vi "POM_PROM_host.vi"() -> ()   [LabVIEW 2013]
uses:
  <instrlib>/niDMM/nidmm.llb/niDMM Resolution in Digits.ctl
  <instrlib>/niDMM/nidmm.llb/niDMM Function.ctl
  <instrlib>/niDCPower/nidcpower.llb/niDCPower Measurement Type.ctl
  <vilib>/Analysis/baseanly.llb/Mean (DBL).vi
  <instrlib>/niDMM/nidmm.llb/niDMM Configure Measurement Digits.vi
  <vilib>/Analysis/NI_AALBase.lvlib
panel:
  in  "Без Офира":bool
  in  "Полярность":bool
  out "Optical Power":dbl(graph)
  out "Operating Current":dbl(graph)=49.97619998441659
  in  "№#":i16=2004
  out "Стабилизировано":bool=TRUE
  in  "+ V TEC для новой точки":dbl=0.11 format="%#_13g"
  in  "Вычет для \"антиразгона\"":dbl format="%#_13g"
  in  "Оставить в раб.\nрежиме":bool
  out "Boolean":bool
  in  "Num_hits_req":u64=5
  out "Num_hits":u64=6
  in  "Count_hits?":bool
  in  "tstab между точками, мс":u32=1
  in  "Предел тока PDext, мА":dbl=20.0
  in  "Dose":i32=1
  in  "Отладка(F)/\n/Рабочий(T)":bool=TRUE
  out "TEC_current, mA":dbl=91.96261106356566
  out "V2(Ild)_Log_address":refnum<file>
  out "Ipd(Ild)_External_Log_address":refnum<file>
  in  "Param_Log":path=path "D:/#rkm/Испытания/Фонон-4/ТермоЛазер/Фонон-4_ПОМ_ПрОМ/Прога/Updated/ThermoLaser/Logs/Добор дозы"
  out "Param_Log_address":refnum<file>
  out "Op(Ild)_Log_address":refnum<file>
  out "Ipd(Ild)_Monitor_Log_address":refnum<file>
  in  "trelax":u32=35000
  out "Volt_onRes":dbl=2.704172165675047
  out "NoStab":bool
  out "Operating Current, mA":dbl=49.97619998441659
  in  "Desirable Operating current, mA":dbl=50.0 format="%#_6f"
  out "Error message":string
  in  "Up_Volt_limit":dbl=5.0
  in  "Low_Volt_limit":dbl=1.0
  out "ThRes_stabil":bool=TRUE
  out "Подстроенное напряжение\nстабилизации":dbl=0.23473322916666667
  out "ThRes value":dbl=17940.031640625
  in  "Optimum ThRes":dbl=18000.0 format="%#_6f"
  in  "Предел тока LD, мА":dbl=80.0
  in  "Предел тока ТЕС, мА":dbl=300.0
  in  "Tab Control":enum32{"Page 1", "Page 2", "Page 3", "Page 4"}(tab)=enum."Page 4"
  out "RES(U_TEC) Graph":cluster{dbl[], dbl[]}(graph)={[-0.0, 0.025, 0.05, 0.07500000000000001, 0.1, 0.125, 0.15, 0.175, 0.19999999999999998, 0.22499999999999998, 0.24999999999999997, 0.27499999999999997, 0.3, 0.325, 0.35000000000000003, 0.37500000000000006, 0.4000000000000001, 0.4250000000000001, 0.4500000000000001, 0.47500000000000014, 0.5000000000000001, 0.5250000000000001, 0.5500000000000002, 0.5750000000000002, 0.6000000000000002, 0.6250000000000002, 0.6500000000000002, 0.6750000000000003, 0.7000000000000003, 0.7250000000000003, 0.7500000000000003, 0.7750000000000004], [15319.04365234375, 15328.19267578125, 15358.49169921875, 15409.562109375, 15479.3826171875, 15563.1861328125, 15668.50888671875, 15780.12734375, 15906.40224609375, 16043.244921875, 16186.97255859375, 16341.84609375, 16507.0697265625, 16676.522265625, 16856.963671875, 17044.884375, 17239.0294921875, 17436.3736328125, 17641.744140625, 17850.8728515625, 18071.7896484375, 18291.20625, 18518.965625, 18750.4271484375, 18987.4517578125, 19230.0744140625, 19480.026171875, 19731.8517578125, 19984.940234375, 20249.54140625, 20514.206640625, 20780.055078125]}
  out "RES(I_TEC) Graph":cluster{dbl[], dbl[]}(graph)={[0.03457500435386299, 4.049114950716204, 7.9212407853678135, 11.611043015146826, 15.078954849250364, 18.53827902856892, 21.88408259580828, 25.295266856430793, 28.546483256934756, 31.60504570629327, 34.77027313644012, 37.80993408960394, 40.856486299311584, 43.94949565069024, 47.03219408159836, 50.06845592920464, 52.92926046093485, 55.95350027659507, 58.865931959242474, 61.84202368829837, 64.7802788203752, 67.60156326899994, 70.44177990185035, 73.41963022613506, 76.46974363403558, 79.22741287887104, 82.2001312992484, 85.07135997639818, 88.0785044464861, 90.98931976346292, 93.95691599392462, 96.75420696595256], [15319.04365234375, 15328.19267578125, 15358.49169921875, 15409.562109375, 15479.3826171875, 15563.1861328125, 15668.50888671875, 15780.12734375, 15906.40224609375, 16043.244921875, 16186.97255859375, 16341.84609375, 16507.0697265625, 16676.522265625, 16856.963671875, 17044.884375, 17239.0294921875, 17436.3736328125, 17641.744140625, 17850.8728515625, 18071.7896484375, 18291.20625, 18518.965625, 18750.4271484375, 18987.4517578125, 19230.0744140625, 19480.026171875, 19731.8517578125, 19984.940234375, 20249.54140625, 20514.206640625, 20780.055078125]}
  out "I_PD_Ext(I_LD) Graph":cluster{dbl[], dbl[]}(graph)={[0.0, 5.125820672560687, 10.202363077068034, 15.09070291650038, 20.026524721844005, 24.848748653112324, 29.706585438813228, 34.55255888002156, 39.41379829521783, 44.31743313126964, 49.35841653002704], [0.6213749657825949, 0.6126206411732633, 0.5986137214569519, 0.5846068013204628, 0.5933611264550083, 0.5670981505590477, 0.5355825775341941, 0.586357666360488, 0.5355825775341941, 0.5478386339632713, 0.5390843079753067]}
  out "I_PD(I_LD) Graph":cluster{dbl[], dbl[]}(graph)={[0.0, 5.125820672560687, 10.202363077068034, 15.09070291650038, 20.026524721844005, 24.848748653112324, 29.706585438813228, 34.55255888002156, 39.41379829521783, 44.31743313126964, 49.35841653002704], [0.00446055423708458, 0.1890051237296575, 1.3185992656872259, 47.69851657329127, 96.3842059718445, 145.3466946259141, 195.95923949964345, 243.1108383461833, 288.08951028622687, 334.6654470078647, 377.8655605856329]}
  out "I_pd, uA":dbl
  out "IPD(ext), mA":dbl
  out "V2(I_LD) Graph":cluster{dbl[], dbl[]}(graph)={[0.0, 5.125820672560687, 10.202363077068034, 15.09070291650038, 20.026524721844005, 24.848748653112324, 29.706585438813228, 34.55255888002156, 39.41379829521783, 44.31743313126964, 49.35841653002704], [0.0006418486043783589, 1.1699665507043246, 1.452329111789965, 1.6798119558569469, 1.9201177244634586, 2.150803801269446, 2.3862573437846697, 2.612869753183121, 2.8439823589319366, 3.0683008415602466, 3.3013683877429134]}
  out "Forward Voltage, V":dbl
  out "OP(I_LD) Graph":cluster{dbl[], dbl[]}(graph)={[0.0, 5.125820672560687, 10.202363077068034, 15.09070291650038, 20.026524721844005, 24.848748653112324, 29.706585438813228, 34.55255888002156, 39.41379829521783, 44.31743313126964, 49.35841653002704], [0.0, 0.0, 0.02, 0.74, 1.5, 2.27, 3.0300000000000002, 3.8, 4.58, 5.33, 6.119999999999999]}
  out "Ophir, mW":dbl
  out "Пороговый ток":dbl
  out "Boolean 2":bool
  out "Сопротивление терморез-ра":dbl(graph)=16035.80078125
  out "thRes_adj":dbl=16035.80078125 format="%0.2f"
  in  "Source-Ohm w8":u32=1000
  in  "Coeff_High":dbl=90000.0 format="%#_13g"
  in  "Coeff_low":dbl=20000.0 format="%#_13g"
  in  "Coeff_thr":dbl=1500.0
  out "+Voltage\nrequired":dbl=0.0008410915798611111
  out "Разница ThRes":dbl=75.6982421875
  out "IPD_ext, mA":dbl(graph)=16035.80078125
  out "accommodated voltage (out)":dbl=5.970992601042338
  in  "4070_Rele_source":enum16{"S2_Ch0", "S1_Ch2"}(ring)
  in  "the upper limit for the voltage_LD":dbl=6.0
  in  "the lower limit for the voltage_LD":dbl=1.0
  in  "Start voltage_LD":dbl=1.5 format="%#.7f"
  in  "accuracy_LD":dbl=0.01 step=0.01
  in  "Res_LD":dbl=50.0
  out "#Итерации":i32=31
  in  "TEC_Source":enum16{"S1_Ch2", "S2_Ch0", "S3_Ch1"}(ring)
  in  "Start voltage":dbl=0.1 format="%#.7f"
  in  "the upper limit for the voltage":dbl=1.0
  in  "the lower limit for the voltage":dbl
  in  "Точность ThRes":dbl=75.0 step=0.01
  out "Ro, Ом":dbl=15321.56484375
  in  "OphirLMMeasurementLib.ICoLMMeasurement":refnum<k7>
  out "hDevice":i32=1000
  out "Ophir_address":refnum<k7>
  in  "Power Enable":bool
  in  "4071(2)":refnum<k15>="PXI1Slot4_2"
  out "4071(2)_adress":refnum<k15>="PXI1Slot4_2 (12)" caption="4071(1)_out"
  in  "4071(1)":refnum<k15>="PXI1Slot5_2"
  out "4071(1)_adress":refnum<k15>="PXI1Slot5_2 (1)" caption="4071(1)_out"
  out "4070_address":refnum<k15>="PXI1Slot6_5 (1)" caption="4070_out"
  in  "4070":refnum<k15>="PXI1Slot6_5"
  in  "Source_3":refnum<k15>
  out "Source_3_Vcc_out":refnum<k15> caption="S_3_out"
  out "Source_2_Vcc_out":refnum<k15>="PXI1Slot3" caption="S_2_out"
  in  "Source_2":refnum<k15>="PXI1Slot3"
  out "Source_1_Vcc_out":refnum<k15>="PXI1Slot2_2" caption="S_1_out"
  in  "Source_1":refnum<k15>="PXI1Slot2_2"
  out "Прервать":bool=TRUE
  in  "milliseconds to wait":u32=2000
  in  "Шаг напр\nдля TEC, В":dbl=0.025
  in  "Начальное\nнапряжение TEC, В":dbl
  in  "кол-во точек для TEC":i32=32
  in  "stop":bool
  in  "Case":T1(ring)=enum."Quit"
  out "Выполняется":bool
  in  "Раб. режим LD":bool
  in  "Хар-ка TEC":bool
  in  "Хар-ки от I_LD":bool
  out "Status:":string="IDLE"
  out "Подстроенный ток, mA":dbl
  in  "Шаг, мА":dbl=5.0
  in  "Начальный ток, мА":dbl
  in  "Кол-во точек":i32=12
  # "20"
  # "7"
  # "5"
  # "0,15"
  # "ток Пельтье во время стабилизации"
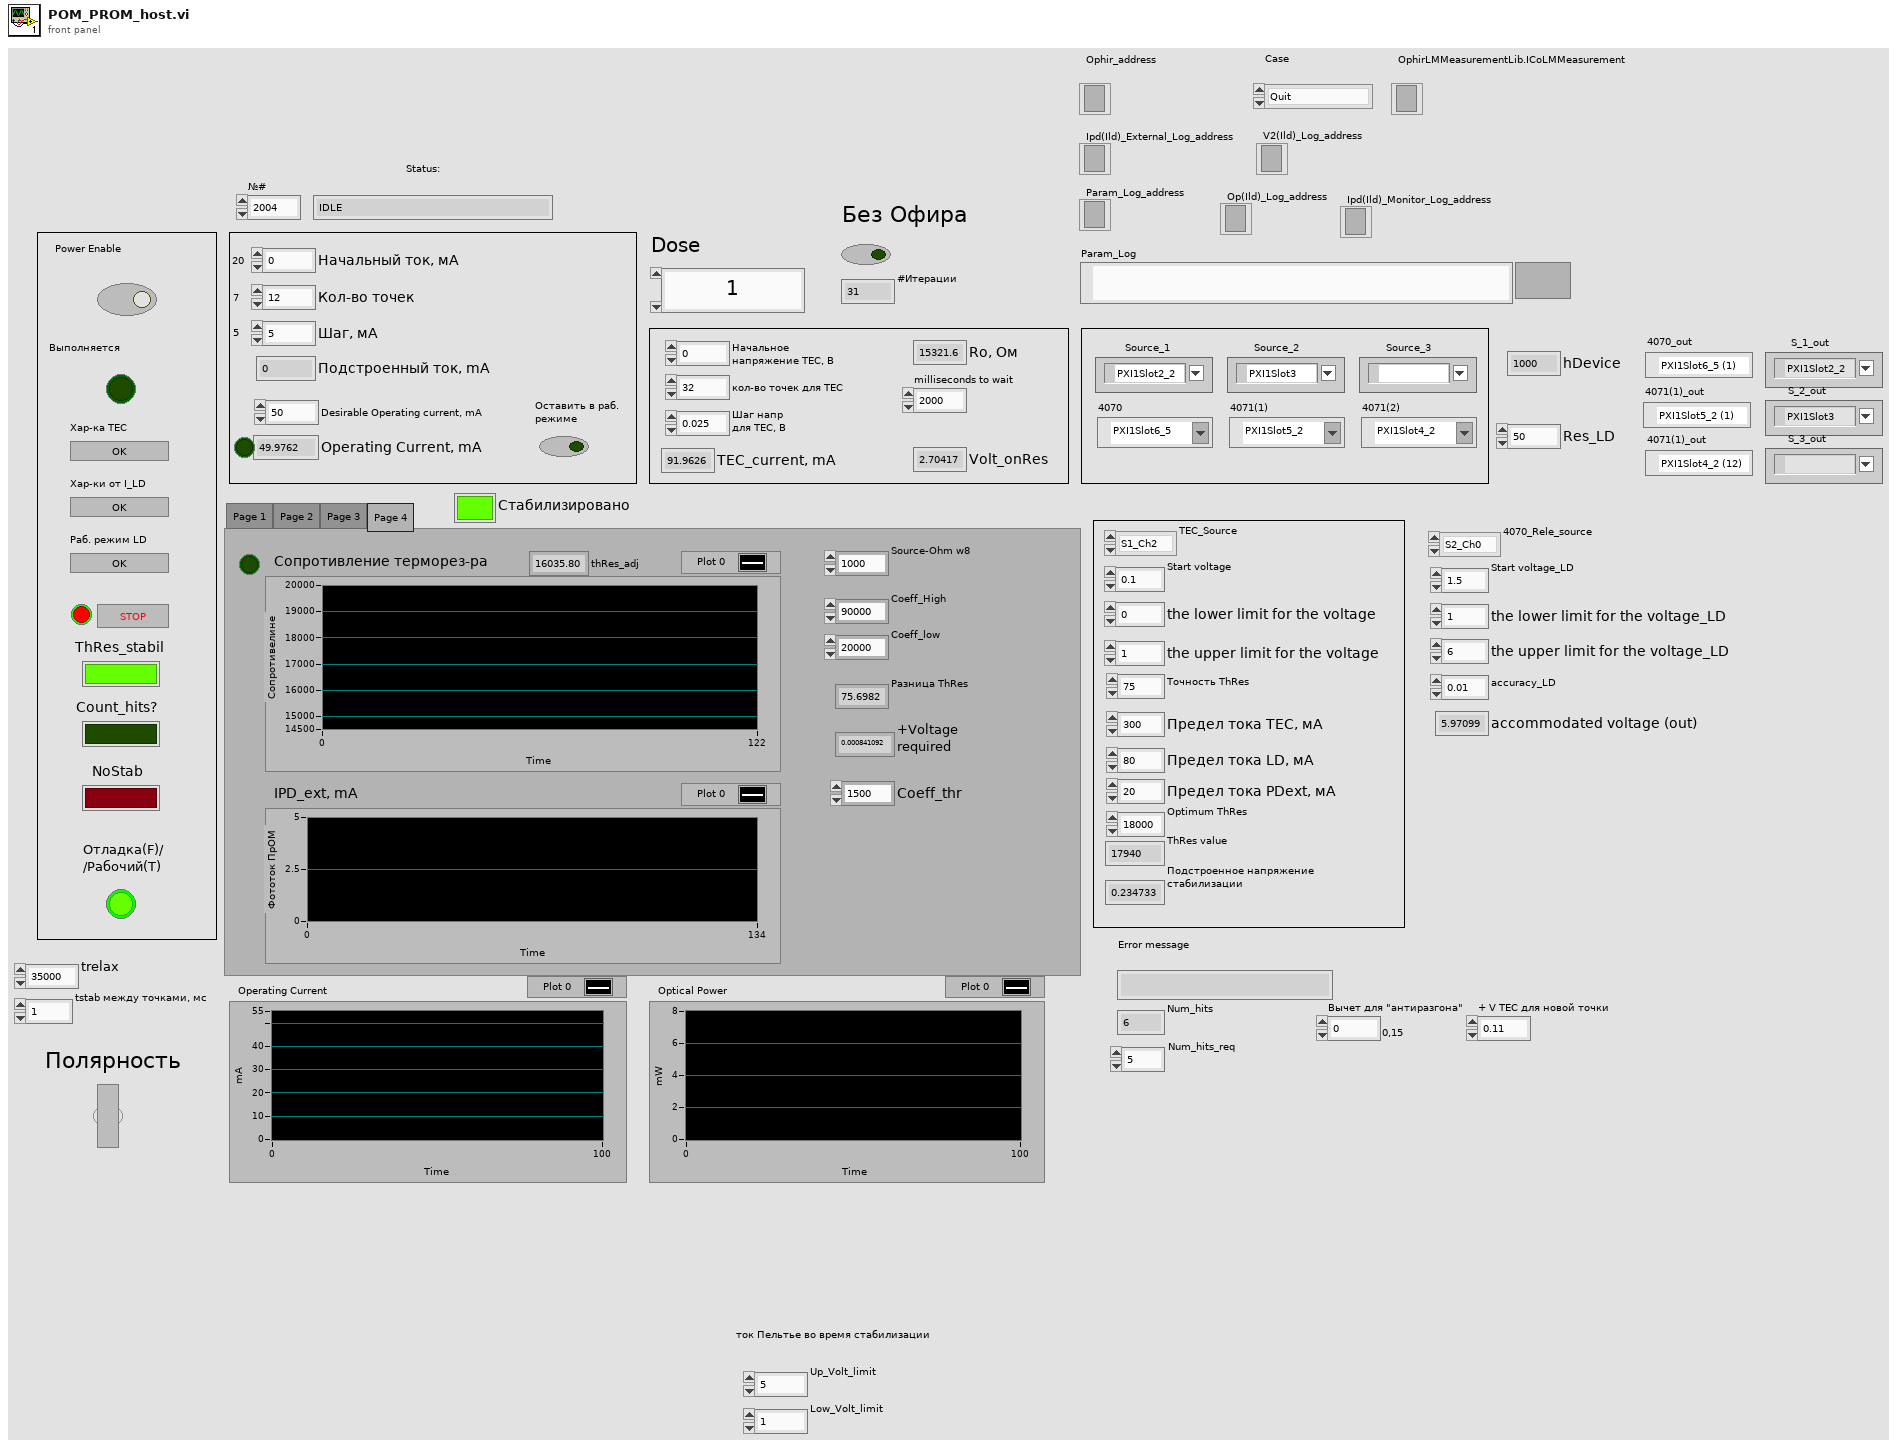
[diagram p1: front panel]
types:
  T1 = enum16{"Initialization", "TEC_Chars", "TRes_Check(Idle)", "Characteristics", "Bias", "Quit"}
  T2 = typedef "niDMM Function.ctl" = enum16{"DC Volts", "AC Volts", "DC Current", "AC Current", "2-wire Resistance", "4-wire Resistance", "Diode", "Frequency", "Period", "AC Volts DC Coupled", "Capacitance", "Inductance", "Temperature"}
  T3 = enum8{"Enabled", "Disabled", "Disabled and Grayed Out"}
  T4 = typedef "niDMM Resolution in Digits.ctl" = dbl
  T5 = enum16{"open", "replace", "create", "open or create", "replace or create", "replace or create with confirmation"}
  T6 = typedef "niDCPower Measurement Type.ctl" = i32
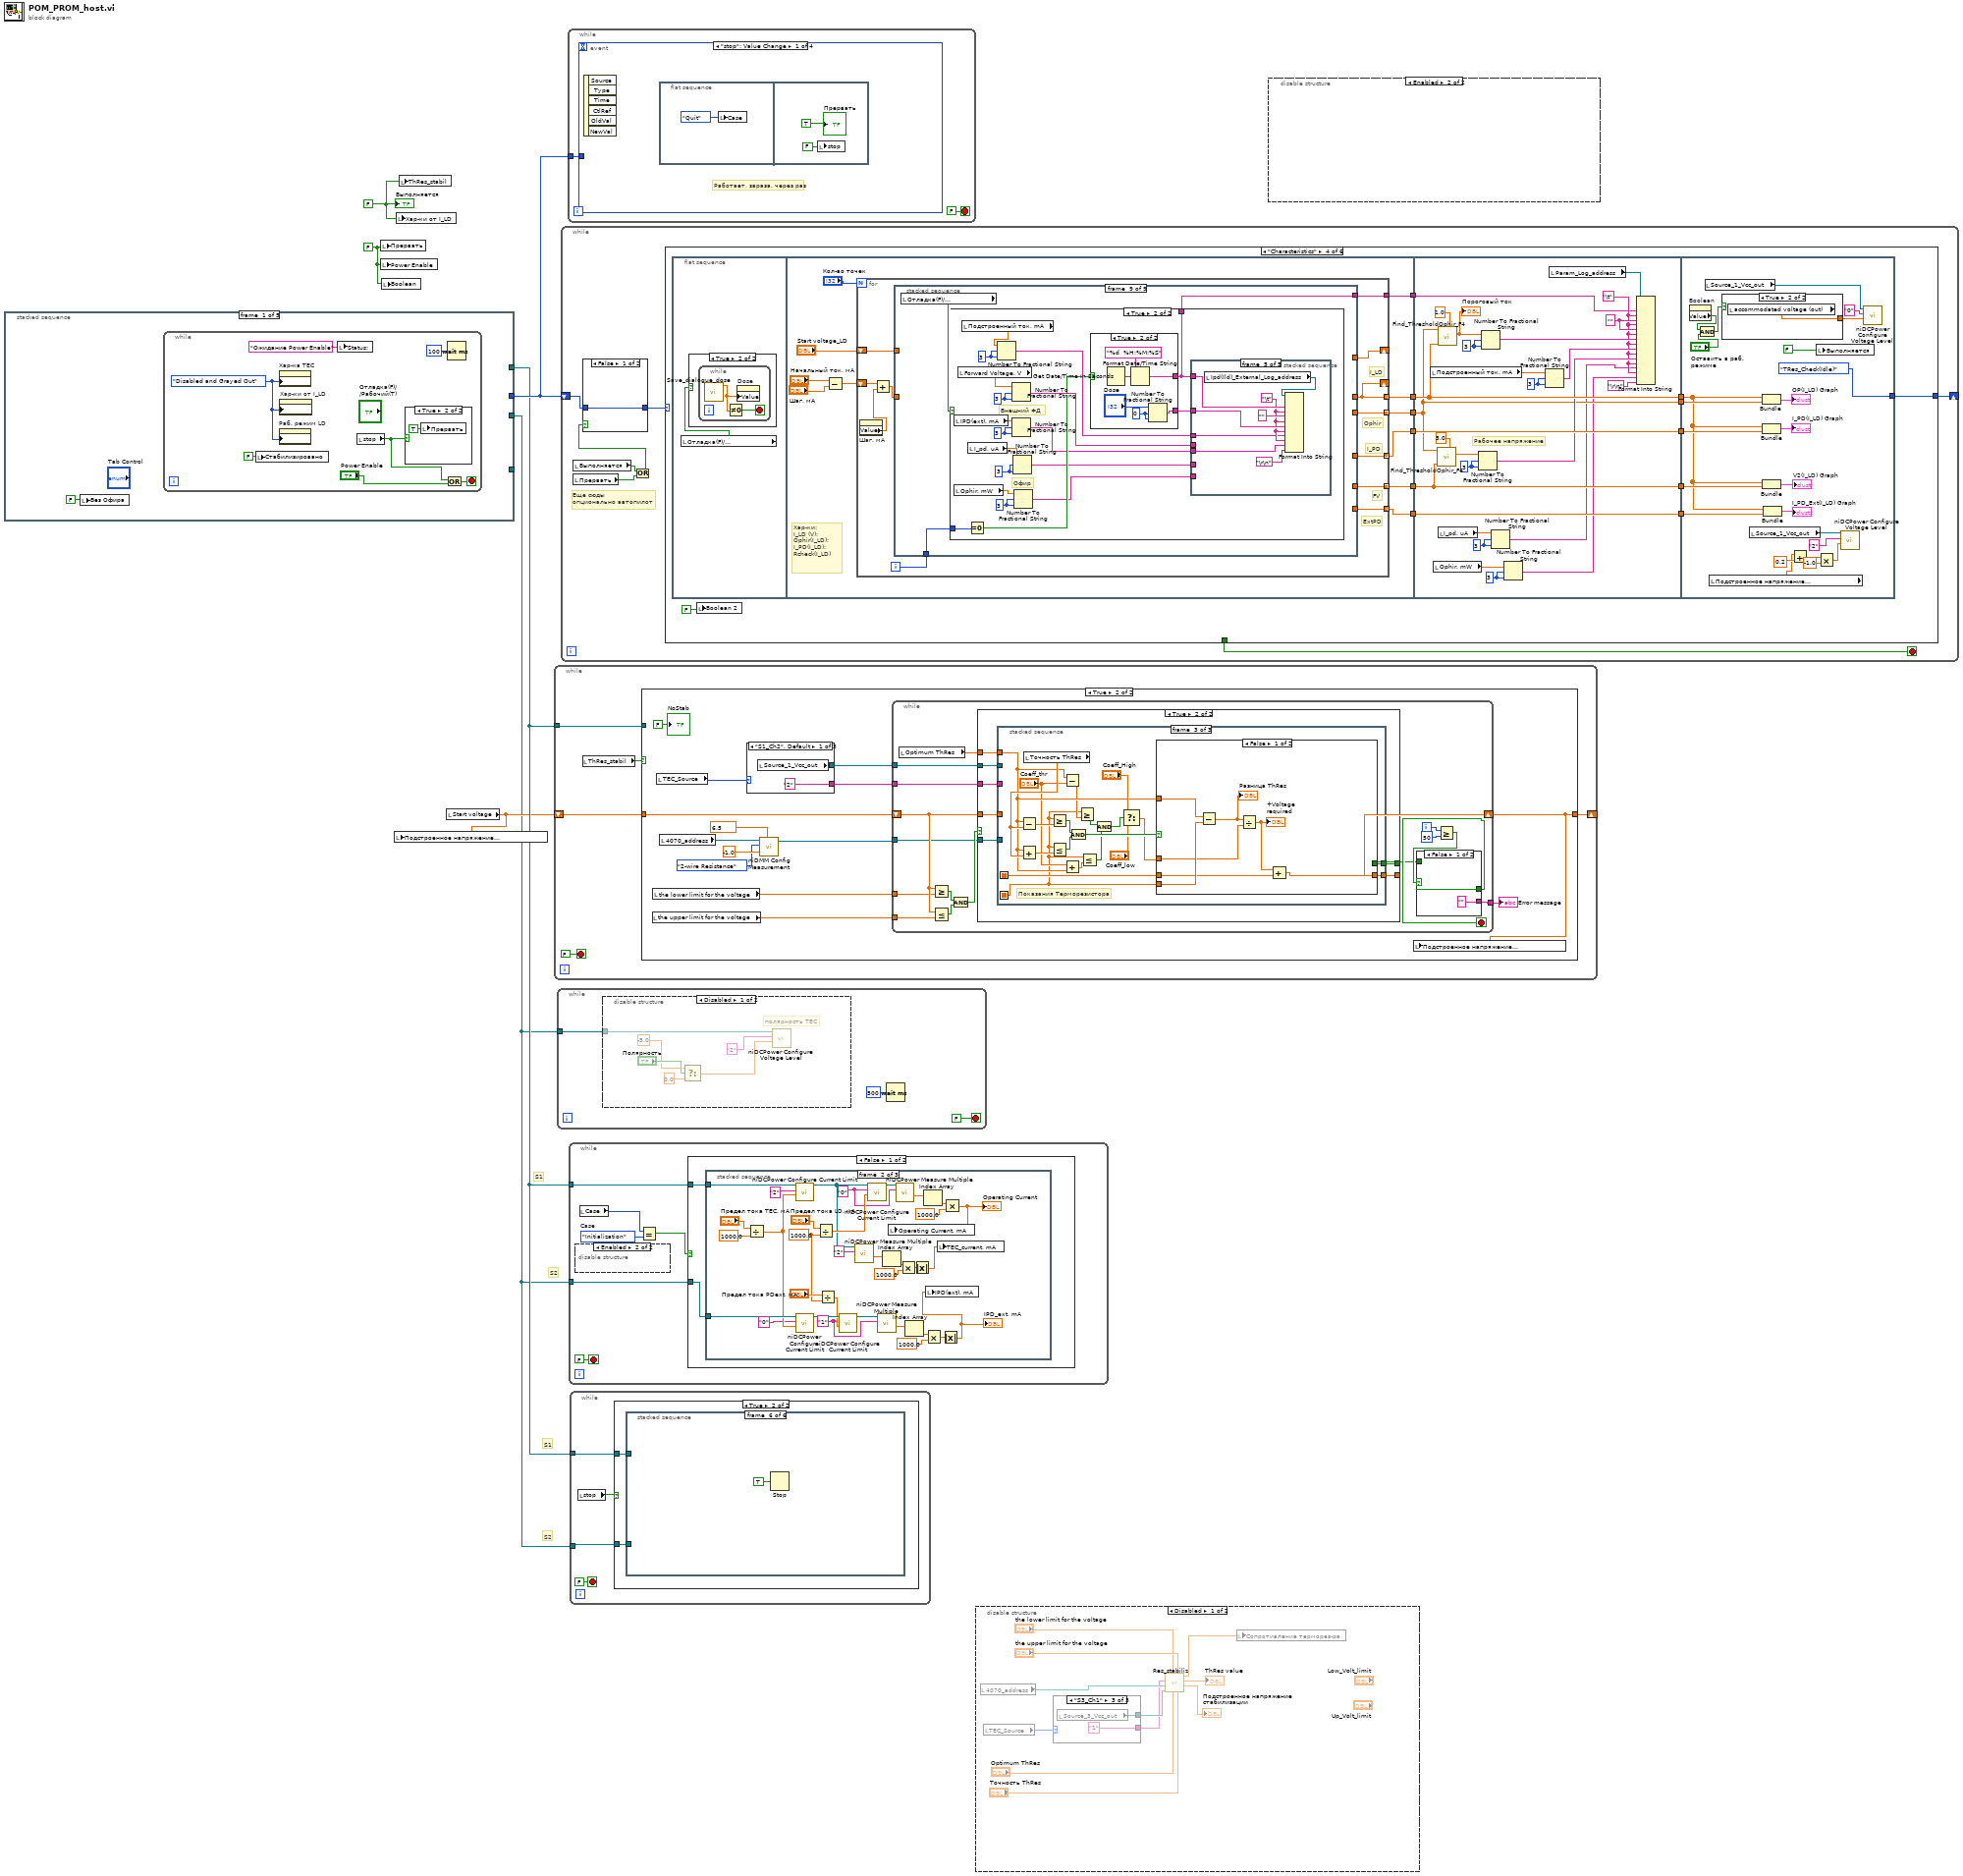
[diagram p0: block diagram]
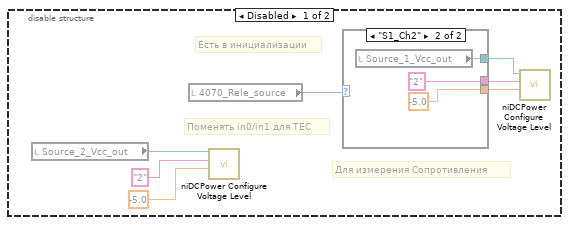
[diagram p3: hidden frame]
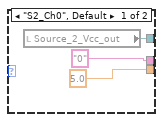
[diagram p4: hidden frame]
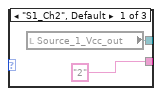
[diagram p5: hidden frame]
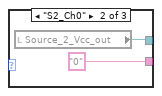
[diagram p6: hidden frame]
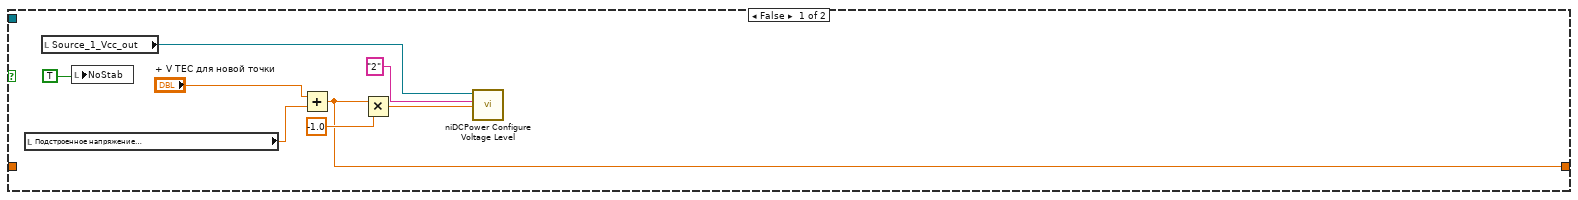
[diagram p8: hidden frame]
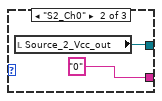
[diagram p9: hidden frame]
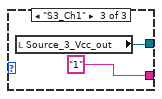
[diagram p10: hidden frame]
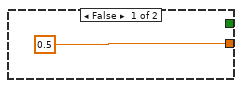
[diagram p11: hidden frame]
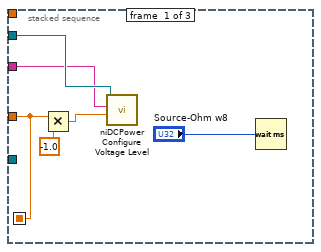
[diagram p12: hidden frame]
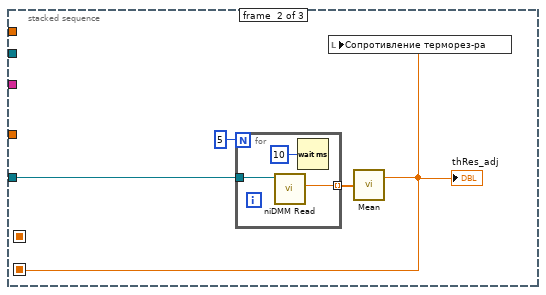
[diagram p13: hidden frame]
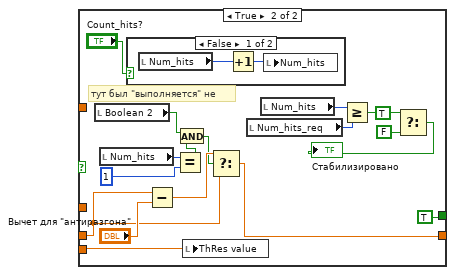
[diagram p14: hidden frame]
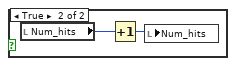
[diagram p15: hidden frame]
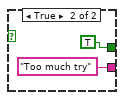
[diagram p16: hidden frame]
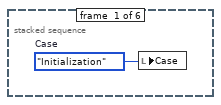
[diagram p18: hidden frame]
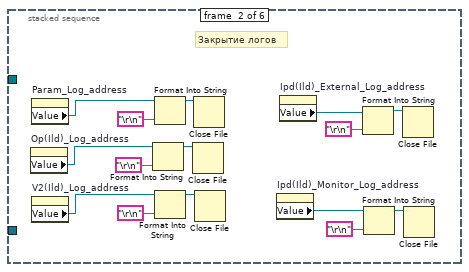
[diagram p19: hidden frame]
diagram:
  w5 = FALSE
  w3 = FALSE
  # "S1"
  # "S2"
  # "S2"
  # "S1"
  n1 = stacked-sequence {
    tunnel: [_ _ _ _ w85] -> w6
    tunnel: [_ w18 _ _ _] -> w1
    tunnel: [_ w17 _ _ _] -> w4
    tunnel: [_ w16 _ _ _] -> _
    frame #0 {
      n2 = local write "Без Офира"(FALSE ("Без Офира")) -> ()
      n3 = while {
        stop <- w14 stop-if-true
        w9 = T3."Disabled and Grayed Out" ("Disabled")
        n4 = local write "Стабилизировано"(FALSE) -> ()
        n5 = property on="Хар-ка TEC" class="Bool (strict)"("DisabledEnum"=w9) -> ()  [unwired: 2 in, 2 out]
        n6 = property on="Раб. режим LD" class="Bool (strict)"("DisabledEnum"=w9) -> ()  [unwired: 2 in, 2 out]
        n7 = property on="Хар-ки от I_LD" class="Bool (strict)"("DisabledEnum"=w9) -> ()  [unwired: 2 in, 2 out]
        n8 = local write "Status:"("Ожидание Power Enable" ("Status:")) -> ()
        n9 = local read "stop"() -> (w12:bool)
        n10 = case shown="True" w12 {
          frame False {
          }
          frame True {
            n11 = local write "Прервать"(TRUE) -> ()
          }
        }
        n12 = Or(x=w12, y="Power Enable") -> (x .or. y?=w14:bool)
        n13 = Wait (ms)(milliseconds to wait=u32 100) -> ()  [unwired: 1 out]
      }
    }
    frame #1 {
      # "Источники"
      n14 = disable-structure shown="Enabled" {
        disable-tunnel: [w39 _] -> w16
        frame Disabled {
          n15 = call <instrlib>:"niDCPower Initialize.vi"("resource name"="Source_3") -> ("instrument handle out"=w43:refnum<k15>)  [unwired: 3 in, 7 out]
          n16 = call <instrlib>:"niDCPower Configure Voltage Level.vi"("voltage level"=0.0, "channel name"="0", "instrument handle"=w43) -> ("instrument handle out"=w42:refnum<k15>)  [unwired: 7 in, 1 out]
          n17 = call <instrlib>:"niDCPower Configure Voltage Level.vi"("voltage level"=0.0, "channel name"="1", "instrument handle"=w42) -> ("instrument handle out"=w48:refnum<k15>)  [unwired: 7 in, 1 out]
          n18 = call <instrlib>:"niDCPower Configure Voltage Level.vi"("voltage level"=0.0, "channel name"="2", "instrument handle"=w48) -> ("instrument handle out"=w39:refnum<k15>)  [unwired: 7 in, 1 out]
          "Source_3_Vcc_out" <- w39
        }
        frame Enabled {
        }
      }
      n19 = call <instrlib>:"niDCPower Initialize.vi"("resource name"="Source_1") -> ("instrument handle out"=w32:refnum<k15>)  [unwired: 3 in, 7 out]
      n20 = call <instrlib>:"niDCPower Initialize.vi"("resource name"="Source_2") -> ("instrument handle out"=w25:refnum<k15>)  [unwired: 3 in, 7 out]
      n21 = call <instrlib>:"niDCPower Configure Voltage Level.vi"("voltage level"=0.0, "channel name"="0", "instrument handle"=w32) -> ("instrument handle out"=w31:refnum<k15>)  [unwired: 7 in, 1 out]
      n22 = call <instrlib>:"niDCPower Configure Voltage Level.vi"("voltage level"=0.0, "channel name"="0", "instrument handle"=w25) -> ("instrument handle out"=w26:refnum<k15>)  [unwired: 7 in, 1 out]
      n23 = call <instrlib>:"niDCPower Configure Voltage Level.vi"("voltage level"=0.0, "channel name"="1", "instrument handle"=w31) -> ("instrument handle out"=w38:refnum<k15>)  [unwired: 7 in, 1 out]
      n24 = call <instrlib>:"niDCPower Configure Voltage Level.vi"("voltage level"=0.0, "channel name"="1", "instrument handle"=w26) -> ("instrument handle out"=w20:refnum<k15>)  [unwired: 7 in, 1 out]
      n25 = call <instrlib>:"niDCPower Configure Voltage Level.vi"("voltage level"=0.0, "channel name"="2", "instrument handle"=w38) -> ("instrument handle out"=w17:refnum<k15>)  [unwired: 7 in, 1 out]
      "Source_1_Vcc_out" <- w17
      n26 = call <instrlib>:"niDCPower Configure Voltage Level.vi"("voltage level"=0.0, "channel name"="2", "instrument handle"=w20) -> ("instrument handle out"=w18:refnum<k15>)  [unwired: 7 in, 1 out]
      "Source_2_Vcc_out" <- w18
    }
    frame #2 {
      w50 = T4 7.5 items=["3 1/2"=3.5, "4 1/2"=4.5, "5 1/2"=5.5, "6 1/2"=6.5, "7 1/2"=7.5] ("Resolution in Digits")
      w52 = TRUE ("Reset")
      (unwired) enum16{"S1_Ch2", "S2_Ch0", "S3_Ch1"}."S1_Ch2"  # TEC_Source
      w63 = T4 6.5 items=["3 1/2"=3.5, "4 1/2"=4.5, "5 1/2"=5.5, "6 1/2"=6.5, "7 1/2"=7.5] ("Resolution in Digits")
      w61 = TRUE ("Reset")
      # "4065"
      # "4070"
      # "Мультиметры"
      n27 = disable-structure shown="Disabled" {
        frame Disabled {
          w70 = T4 7.5 items=["3 1/2"=3.5, "4 1/2"=4.5, "5 1/2"=5.5, "6 1/2"=6.5, "7 1/2"=7.5] ("Resolution in Digits")
          w68 = TRUE ("Reset")
          # "4071"
          n28 = call <instrlib>:"niDMM Initialize.vi"("Reset"=w68, "ID Query"=w68, "Instrument Descriptor"="4071(2)") -> ("instrument handle out"=w66:refnum<k15>)  [unwired: 7 in, 1 out]
          n29 = call-poly <instrlib>:"niDMM Config Measurement.vi"("Range"=-1.0 ("Configuration:Measurement Options:Max Frequency"), "Resolution in Digits"=w70, "Function"=niDMM_Function."DC Current" ("multimeter mode"), "instrument handle"=w66) -> ("instrument handle out"=w64:refnum<k15>)  [unwired: 6 in, 1 out]
          "4071(2)_adress" <- w64
          n30 = call <instrlib>:"niDMM Read.vi"("instrument handle"=w64) -> ()  [unwired: 8 in, 3 out]
        }
        frame Enabled {
        }
      }
      n31 = call <instrlib>:"niDMM Initialize.vi"("Reset"=w52, "ID Query"=w52, "Instrument Descriptor"="4071(1)") -> ("instrument handle out"=w54:refnum<k15>)  [unwired: 7 in, 1 out]
      n32 = call <instrlib>:"niDMM Initialize.vi"("Reset"=w61, "ID Query"=w61, "Instrument Descriptor"="4070") -> ("instrument handle out"=w59:refnum<k15>)  [unwired: 7 in, 1 out]
      n33 = call-poly <instrlib>:"niDMM Config Measurement.vi"("Range"=-1.0 ("Configuration:Measurement Options:Max Frequency"), "Resolution in Digits"=w50, "Function"=niDMM_Function."DC Current" ("multimeter mode"), "instrument handle"=w54) -> ("instrument handle out"=→"4071(1)_adress":refnum<k15>)  [unwired: 6 in, 1 out]
      n34 = call-poly <instrlib>:"niDMM Config Measurement.vi"("Range"=-1.0 ("Configuration:Measurement Options:Max Frequency"), "Resolution in Digits"=w63, "Function"=niDMM_Function."DC Current" ("multimeter mode"), "instrument handle"=w59) -> ("instrument handle out"=→"4070_address":refnum<k15>)  [unwired: 6 in, 1 out]
    }
    frame #3 {
      n35 = case shown="False" "Без Офира" {
        frame False {
          n36 = Automation Open(Automation Refnum="OphirLMMeasurementLib.ICoLMMeasurement") -> (Automation Refnum=w80:refnum<k7>)  [unwired: 3 in, 1 out]
          n37 = invoke class="ICoLMMeasurement" method="ScanUSB"(reference=w80) -> (reference out=w82:refnum<k7>, "serialNumbers"=w79:variant)  [unwired: 3 in, 2 out]
          "Ophir_address" <- w82
          n38 = Variant To Data(type=string[] [], Variant=w79) -> (data=w78:string[])  [unwired: 1 in, 1 out]
          n39 = Index Array(array=w78, index=0) -> (element=w75:string)
          n40 = invoke class="ICoLMMeasurement" method="OpenUSBDevice"(reference=w82, "serialNumber"=w75) -> (reference out=w74:refnum<k7>, "hDevice"=w73:i32)  [unwired: 3 in, 3 out]
          "hDevice" <- w73
          n41 = invoke class="ICoLMMeasurement" method="StartStream"(reference=w74, "hDevice"=w73, "channel"=0) -> ()  [unwired: 2 in, 5 out]
        }
        frame True {
        }
      }
    }
    frame #4 {
      (unwired) enum16{"S2_Ch0", "S1_Ch2"}."S2_Ch0"  # 4070_Rele_source
      w85 = T1."Initialization"  # Case
      n42 = disable-structure shown="Disabled" {
        frame Disabled {
          n43 = while {
            stop <- w86 stop-if-true
            n44 = One Button Dialog(message="Ну тут в общем хмм...мда", button name ("OK")="что поделать, продолжаем") -> (true=w86:bool)
          }
        }
        frame Enabled {
        }
      }
      n45 = property on="Сопротивление терморез-ра" class="WFChart (strict)"("History Data"=dbl[] []) -> ()  [unwired: 2 in, 2 out]
      n46 = local write "Start voltage"("Start voltage") -> ()
    }
  }
  n47 = local write "Прервать"(w3) -> ()
  n48 = local write "Power Enable"(w3) -> ()
  n49 = local write "Boolean"(w3) -> ()
  n50 = local write "Хар-ки от I_LD"(w5) -> ()
  n51 = local write "ThRes_stabil"(w5) -> ()
  n52 = local read "Start voltage"() -> (w2:dbl)
  n53 = local write "Подстроенное напряжение\nстабилизации"(w2) -> ()
  n54 = while {
    shift-right: [w91] -> _
    shift-left: w2 -> [w90]
    tunnel: w4 -> [w89]
    stop <- FALSE stop-if-true
    n55 = local read "ThRes_stabil"() -> (w92:bool)
    n56 = case shown="True" w92 {
      tunnel: [w95 w103] -> w91
      tunnel: w90 -> [_ w109]
      tunnel: w89 -> [_ _]
      frame False {
        n57 = local read "Подстроенное напряжение\nстабилизации"() -> (w94:dbl)
        n58 = local read "Source_1_Vcc_out"() -> (w99:refnum<k15>)
        n59 = local write "NoStab"(TRUE) -> ()
        n60 = Add(x="+ V TEC для новой точки", y=w94) -> (x+y=w95:dbl)
        n61 = Multiply(x=w95, y=-1.0) -> (x*y=w96:dbl)
        n62 = call <instrlib>:"niDCPower Configure Voltage Level.vi"("voltage level"=w96, "channel name"="2", "instrument handle"=w99) -> ()  [unwired: 7 in, 2 out]
      }
      frame True {
        w105 = T4 6.5 items=["3 1/2"=3.5, "4 1/2"=4.5, "5 1/2"=5.5, "6 1/2"=6.5, "7 1/2"=7.5] ("Resolution in Digits")
        n63 = local read "the upper limit for the voltage"() -> (w110:dbl)
        n64 = local read "the lower limit for the voltage"() -> (w111:dbl)
        n65 = local read "TEC_Source"() -> (w112:enum16{"S1_Ch2", "S2_Ch0", "S3_Ch1"})
        n66 = local read "4070_address"() -> (w104:refnum<k15>)
        n67 = case shown="\"S1_Ch2\", Default" w112 {
          tunnel: [w117 w119 w121] -> w114
          tunnel: ["2" "0" "1"] -> w113
          frame "S1_Ch2", Default {
            n68 = local read "Source_1_Vcc_out"() -> (w117:refnum<k15>)
          }
          frame "S2_Ch0" {
            n69 = local read "Source_2_Vcc_out"() -> (w119:refnum<k15>)
          }
          frame "S3_Ch1" {
            n70 = local read "Source_3_Vcc_out"() -> (w121:refnum<k15>)
          }
        }
        n71 = call-poly <instrlib>:"niDMM Config Measurement.vi"("Range"=-1.0 ("Configuration:Measurement Options:Max Frequency"), "Resolution in Digits"=w105, "Function"=niDMM_Function."2-wire Resistance" ("multimeter mode"), "instrument handle"=w104) -> ("instrument handle out"=w102:refnum<k15>)  [unwired: 6 in, 1 out]
        n72 = while {
          tunnel: w113 -> [w129]
          tunnel: w114 -> [w130]
          tunnel: w102 -> [w128]
          shift-right: [w127] -> w103
          shift-left: w109 -> [w131]
          tunnel: [w125] -> w115
          tunnel: w111 -> [w123]
          tunnel: w110 -> [w122]
          i -> [w135]
          stop <- w136 stop-if-true
          n73 = local read "Optimum ThRes"() -> (w124:dbl)
          n74 = Greater Or Equal?(x=w131, y=w123) -> (x >= y?=w134:bool)
          n75 = Less Or Equal?(x=w131, y=w122) -> (x <= y?=w133:bool)
          n76 = And(x=w134, y=w133) -> (x .and. y?=w132:bool)
          n77 = case shown="True" w132 {
            tunnel: w131 -> [_ w144]
            tunnel: w130 -> [_ w146]
            tunnel: w129 -> [_ w145]
            tunnel: w124 -> [_ w142]
            tunnel: w128 -> [_ w143]
            tunnel: [0.5 w141] -> w127
            tunnel: [_ w140] -> w126
            frame False {
            }
            frame True {
              n78 = stacked-sequence {
                seq-local: [w147 _ _] -> [_ _ w174]
                seq-local: [_ w154 _] -> [_ _ w164]
                tunnel: w146 -> [w152 _ _]
                tunnel: w145 -> [w151 _ _]
                tunnel: w144 -> [w147 _ _]
                tunnel: w143 -> [_ w153 _]
                tunnel: w142 -> [_ _ w167]
                tunnel: [_ _ w173] -> w141
                tunnel: [_ _ w172] -> w140
                frame #0 {
                  n79 = Multiply(x=w147, y=-1.0) -> (x*y=w148:dbl)
                  n80 = call <instrlib>:"niDCPower Configure Voltage Level.vi"("voltage level"=w148, "channel name"=w151, "instrument handle"=w152) -> ()  [unwired: 7 in, 2 out]
                  n81 = Wait (ms)(milliseconds to wait="Source-Ohm w8") -> ()  [unwired: 1 out]
                }
                frame #1 {
                  n82 = for {
                    N: 5 -> [_]
                    tunnel: w153 -> [w159]
                    tunnel: [w158] -> w155 mode=indexing
                    n83 = call <instrlib>:"niDMM Read.vi"("instrument handle"=w159) -> ("Measurement"=w158:dbl)  [unwired: 8 in, 2 out]
                    n84 = Wait (ms)(milliseconds to wait=u32 10) -> ()  [unwired: 1 out]
                  }
                  n85 = call-poly <vilib>:"Mean.vi"("X"=w155) -> ("mean"=w154:dbl)  [unwired: 1 out]
                  "thRes_adj" <- w154
                  n86 = local write "Сопротивление терморез-ра"(w154) -> ()
                }
                frame #2 {
                  # "Показания Терморезистора"
                  n87 = local read "Точность ThRes"() -> (w171:dbl)
                  n88 = Subtract(x=w167, y=w171) -> (x-y=w177:dbl)
                  n89 = Add(x=w167, y=w171) -> (x+y=w178:dbl)
                  n90 = Greater Or Equal?(x=w164, y=w177) -> (x >= y?=w179:bool)
                  n91 = Less Or Equal?(x=w164, y=w178) -> (x <= y?=w176:bool)
                  n92 = Subtract(x=w167, y="Coeff_thr") -> (x-y=w165:dbl)
                  n93 = Add(x="Coeff_thr", y=w167) -> (x+y=w163:dbl)
                  n94 = And(x=w179, y=w176) -> (x .and. y?=w175:bool)
                  n95 = Greater Or Equal?(x=w164, y=w165) -> (x >= y?=w162:bool)
                  n96 = Less Or Equal?(x=w164, y=w163) -> (x <= y?=w161:bool)
                  n97 = And(x=w162, y=w161) -> (x .and. y?=w160:bool)
                  n98 = Select(t="Coeff_High", s=w160, f="Coeff_low") -> (s? t:f=w168:dbl)
                  n99 = case shown="False" w175 {
                    tunnel: [w181 w196] -> w173
                    tunnel: w174 -> [w183 w197]
                    tunnel: [_ TRUE] -> w172
                    tunnel: w164 -> [w184 w203]
                    tunnel: w167 -> [w185 _]
                    tunnel: w168 -> [w180 _]
                    frame False {
                      n100 = Subtract(x=w185, y=w184) -> (x-y=w186:dbl)
                      "Разница ThRes" <- w186
                      n101 = Divide(x=w186, y=w180) -> (x/y=w182:dbl)
                      "+Voltage\nrequired" <- w182
                      n102 = Add(x=w182, y=w183) -> (x+y=w181:dbl)
                    }
                    frame True {
                      # "тут был \"выполняется\" не"
                      n103 = local read "Boolean 2"() -> (w187:bool)
                      n104 = local read "Num_hits"() -> (w201:u64)
                      n105 = case shown="False" "Count_hits?" {
                        frame False {
                          n106 = local read "Num_hits"() -> (w205:u64)
                          n107 = Increment(x=w205) -> (x+1=w206:u64)
                          n108 = local write "Num_hits"(w206) -> ()
                        }
                        frame True {
                          n109 = local read "Num_hits"() -> (w208:u64)
                          n110 = Increment(x=w208) -> (x+1=w207:u64)
                          n111 = local write "Num_hits"(w207) -> ()
                        }
                      }
                      n112 = Subtract(x=w197, y="Вычет для \"антиразгона\"") -> (x-y=w198:dbl)
                      n113 = Equal?(x=w201, y=1) -> (x = y?=w195:bool)
                      n114 = And(x=w187, y=w195) -> (x .and. y?=w194:bool)
                      n115 = local write "ThRes value"(w203) -> ()
                      n116 = Select(t=w198, s=w194, f=w197) -> (s? t:f=w196:dbl)
                      n117 = local read "Num_hits_req"() -> (w192:u64)
                      n118 = local read "Num_hits"() -> (w193:u64)
                      n119 = Greater Or Equal?(x=w193, y=w192) -> (x >= y?=w191:bool)
                      n120 = Select(t=TRUE, s=w191, f=FALSE) -> (s? t:f=→"Стабилизировано":bool)
                    }
                  }
                }
              }
            }
          }
          n121 = Greater Or Equal?(x=w135, y=50) -> (x >= y?=w137:bool)
          n122 = case shown="False" w137 {
            tunnel: ["" "Too much try"] -> w125
            tunnel: [w210 TRUE] -> w136
            tunnel: w126 -> [w210 _]
            frame False {
            }
            frame True {
            }
          }
        }
        "Error message" <- w115
        n123 = local write "Подстроенное напряжение\nстабилизации"(w103) -> ()
        "NoStab" <- FALSE ("NoStab")
      }
    }
  }
  n124 = while {
    tunnel: w1 -> [w213]
    stop <- FALSE stop-if-true
    n125 = disable-structure shown="Disabled" {
      disable-tunnel: w213 -> [w216 _]
      frame Disabled {
        # "полярность ТЕС"
        n126 = Select(t=-5.0, s="Полярность", f=0.0) -> (s? t:f=w217:dbl)
        n127 = call <instrlib>:"niDCPower Configure Voltage Level.vi"("voltage level"=w217, "channel name"="2", "instrument handle"=w216) -> ()  [unwired: 7 in, 2 out]
      }
      frame Enabled {
      }
    }
    n128 = Wait (ms)(milliseconds to wait=u32 500) -> ()  [unwired: 1 out]
  }
  n129 = while {
    shift-right: [w222] -> _
    shift-left: w6 -> [w228]
    stop <- w226 stop-if-true
    # "Еще сюды\nопционально автопилот"
    n130 = local read "Выполняется"() -> (w225:bool)
    n131 = local read "Прервать"() -> (w224:bool)
    n132 = Or(x=w225, y=w224) -> (x .or. y?=w223:bool)
    n133 = case shown="False" w223 {
      tunnel: w228 -> [w229 _]
      tunnel: [w229 "Case"] -> w227
      frame False {
      }
      frame True {
      }
    }
    n134 = case shown="\"Characteristics\"" w227 {
      tunnel: [_ _ _ _ _ TRUE] -> w226
      tunnel: [w231 w358 w527 w567 w848 T1."Quit" ("Case")] -> w222
      frame "Initialization", Default {
        n135 = stacked-sequence {
          tunnel: [_ _ _ _ T1."TRes_Check(Idle)" ("Case")] -> w231
          frame #0 {
            w234 = T3."Enabled" ("Disabled")
            n136 = property on="Хар-ка TEC" class="Bool (strict)"("DisabledEnum"=w234) -> ()  [unwired: 2 in, 2 out]
            n137 = property on="Раб. режим LD" class="Bool (strict)"("DisabledEnum"=w234) -> ()  [unwired: 2 in, 2 out]
            n138 = property on="Хар-ки от I_LD" class="Bool (strict)"("DisabledEnum"=w234) -> ()  [unwired: 2 in, 2 out]
          }
          frame #1 {
            # "Питание внешнего фотодиода"
            # "Поменять in0/in1 для ТЕС"
            # "Режим омметра"
            n139 = local read "4070_Rele_source"() -> (w242:enum16{"S2_Ch0", "S1_Ch2"})
            n140 = local read "Source_2_Vcc_out"() -> (w240:refnum<k15>)
            n141 = local read "Source_2_Vcc_out"() -> (w237:refnum<k15>)
            n142 = case shown="\"S2_Ch0\", Default" w242 {
              tunnel: [5.0 -5.0] -> w243
              tunnel: ["0" "2"] -> w244
              tunnel: [w246 w249] -> w245
              frame "S2_Ch0", Default {
                n143 = local read "Source_2_Vcc_out"() -> (w246:refnum<k15>)
              }
              frame "S1_Ch2" {
                n144 = local read "Source_1_Vcc_out"() -> (w249:refnum<k15>)
              }
            }
            n145 = call <instrlib>:"niDCPower Configure Voltage Level.vi"("voltage level"=-5.0, "channel name"="2", "instrument handle"=w240) -> ()  [unwired: 7 in, 2 out]
            n146 = call <instrlib>:"niDCPower Configure Voltage Level.vi"("voltage level"=5.0, "channel name"="1", "instrument handle"=w237) -> ()  [unwired: 7 in, 2 out]
            n147 = call <instrlib>:"niDCPower Configure Voltage Level.vi"("voltage level"=w243, "channel name"=w244, "instrument handle"=w245) -> ()  [unwired: 7 in, 2 out]
            n148 = Wait (ms)(milliseconds to wait=u32 500) -> ()  [unwired: 1 out]
          }
          frame #2 {
            w254 = FALSE
            n149 = local write "NoStab"(w254) -> ()
            n150 = local write "Count_hits?"(w254) -> ()
            n151 = local write "Num_hits"(u64 0 ("Num_hits")) -> ()
            "ThRes_stabil" <- TRUE
            "Boolean 2" <- TRUE
          }
          frame #3 {
            w267 = "\t"
            w283 = "\t"
            w339 = "\t"
            w343 = "\t"
            w300 = "\t"
            n152 = Number To Fractional String(number="№#", width (-)=i16 1, precision (6)=i16 0) -> (F-format string=w275:string)  [unwired: 1 in]
            n153 = Build Path(base path="Param_Log", name or relative path=w275) -> (appended path=w310:path)
            n154 = call <vilib>:"Check if File or Folder Exists.vi"("path"=w310) -> ("file or folder exists?"=w308:bool, "dup path"=w309:path)  [unwired: 8 in, 1 out]
            n155 = Concatenate Strings(w275, "_" ("element"), "Param_log" ("string"), ".txt" ("element")) -> (w304:string)
            n156 = Concatenate Strings(w275, "_" ("element"), "Op(Ild)_log" ("string"), ".txt" ("element")) -> (w319:string)
            n157 = Concatenate Strings(w275, "_" ("element"), "Ipd(Ild)_Monitor_log" ("string"), ".txt" ("element")) -> (w330:string)
            n158 = Concatenate Strings(w275, "_" ("element"), "Ipd(Ild)_External_log" ("string"), ".txt" ("element")) -> (w289:string)
            n159 = Concatenate Strings(w275, "_" ("element"), "V2(Ild)_log" ("string"), ".txt" ("element")) -> (w271:string)
            n160 = case shown="False" w308 {
              tunnel: w309 -> [w355 w356]
              tunnel: [w354 w356] -> w260
              frame False {
                n161 = Create Folder(path (use dialog)=w355) -> (created path=w354:path)  [unwired: 2 in, 2 out]
              }
              frame True {
              }
            }
            n162 = Build Path(base path=w260, name or relative path=w304) -> (appended path=w305:path)
            n163 = Build Path(base path=w260, name or relative path=w271) -> (appended path=w273:path)
            n164 = Build Path(base path=w260, name or relative path=w319) -> (appended path=w321:path)
            n165 = Build Path(base path=w260, name or relative path=w330) -> (appended path=w325:path)
            n166 = Build Path(base path=w260, name or relative path=w289) -> (appended path=w291:path)
            n167 = Open/Create/Replace File(file path (use dialog)=w305, operation (0:open)=T5."open or create", access (0:read/write)=enum16{"read/write", "read-only", "write-only"}."read/write") -> (refnum out=w298:refnum<file>)  [unwired: 3 in, 2 out]
            "Param_Log_address" <- w298
            n168 = Open/Create/Replace File(file path (use dialog)=w321, operation (0:open)=T5."open or create", access (0:read/write)=enum16{"read/write", "read-only", "write-only"}."read/write") -> (refnum out=w299:refnum<file>)  [unwired: 3 in, 2 out]
            "Op(Ild)_Log_address" <- w299
            n169 = Open/Create/Replace File(file path (use dialog)=w273, operation (0:open)=T5."open or create", access (0:read/write)=enum16{"read/write", "read-only", "write-only"}."read/write") -> (refnum out=w261:refnum<file>)  [unwired: 3 in, 2 out]
            "V2(Ild)_Log_address" <- w261
            n170 = Open/Create/Replace File(file path (use dialog)=w325, operation (0:open)=T5."open or create", access (0:read/write)=enum16{"read/write", "read-only", "write-only"}."read/write") -> (refnum out=w336:refnum<file>)  [unwired: 3 in, 2 out]
            "Ipd(Ild)_Monitor_Log_address" <- w336
            n171 = Open/Create/Replace File(file path (use dialog)=w291, operation (0:open)=T5."open or create", access (0:read/write)=enum16{"read/write", "read-only", "write-only"}."read/write") -> (refnum out=w279:refnum<file>)  [unwired: 3 in, 2 out]
            "Ipd(Ild)_External_Log_address" <- w279
            n172 = Format Into String(initial string=w298, "Time" ("input 1"), w300, "Mode" ("input 6"), w300, "Dose" ("input 1"), w300, "Thr_Cur, mA" ("input 6"), w300, "Op_Cur, mA " ("input 6"), w300, "Op_Vol, V" ("input 6"), w300, "Ipd, uA" ("input 6"), w300, "OutPow, mW" ("input 6"), w300, "Dark_Cur, uA" ("input 6"), "\r\n") -> (resulting string=w311:refnum<file>)  [unwired: 2 in, 1 out]
            n173 = Format Into String(initial string=w336, "Time" ("input 1"), w339, "Mode" ("input 6"), w339, "Dose" ("input 1"), w339, "Ild, mA" ("input 6"), w339, "Ipd, uA" ("input 6"), w339, "\r\n") -> (resulting string=w333:refnum<file>)  [unwired: 2 in, 1 out]
            n174 = Format Into String(initial string=w261, "Time" ("input 1"), w267, "Mode" ("input 6"), w267, "Dose" ("input 1"), w267, "Ild, mA" ("input 6"), w267, "V2, V" ("input 6"), w267, "\r\n") -> (resulting string=w262:refnum<file>)  [unwired: 2 in, 1 out]
            n175 = Set File Position(refnum=w333, from (0:start)=enum16{"start", "end", "current"}."end") -> ()  [unwired: 2 in, 2 out]
            n176 = Set File Position(refnum=w262, from (0:start)=enum16{"start", "end", "current"}."end") -> ()  [unwired: 2 in, 2 out]
            n177 = Set File Position(refnum=w311, from (0:start)=enum16{"start", "end", "current"}."end") -> ()  [unwired: 2 in, 2 out]
            n178 = Format Into String(initial string=w299, "Time" ("input 1"), w343, "Mode" ("input 6"), w343, "Dose" ("input 1"), w343, "Ild, mA" ("input 6"), w343, "Op, mW" ("input 6"), "\r\n") -> (resulting string=w332:refnum<file>)  [unwired: 2 in, 1 out]
            n179 = Format Into String(initial string=w279, "Time" ("input 1"), w283, "Mode" ("input 6"), w283, "Dose" ("input 1"), w283, "Ild, mA" ("input 6"), w283, "IPD, mA" ("input 6"), w283, "\r\n") -> (resulting string=w288:refnum<file>)  [unwired: 2 in, 1 out]
            n180 = Set File Position(refnum=w332, from (0:start)=enum16{"start", "end", "current"}."end") -> ()  [unwired: 2 in, 2 out]
            n181 = Set File Position(refnum=w288, from (0:start)=enum16{"start", "end", "current"}."end") -> ()  [unwired: 2 in, 2 out]
          }
          frame #4 {
          }
        }
        n182 = Wait (ms)(milliseconds to wait=u32 100) -> ()  [unwired: 1 out]
        "Status:" <- "Инициализация" ("Status:")
      }
      frame "TEC_Chars" {
        n183 = while {
          tunnel: [w360] -> w358
          stop <- w359 stop-if-true
          n184 = stacked-sequence {
            tunnel: [_ _ w406 _] -> w360
            tunnel: [_ _ w404 _] -> w359
            frame #0 {
              n185 = local write "Boolean 2"(FALSE) -> ()
              n186 = stacked-sequence {
                frame #0 {
                  # "Переключение в режим Омметра"
                  n187 = local read "4070_Rele_source"() -> (w366:enum16{"S2_Ch0", "S1_Ch2"})
                  n188 = case shown="\"S2_Ch0\", Default" w366 {
                    tunnel: [5.0 -5.0] -> w365
                    tunnel: ["0" "2"] -> w364
                    tunnel: [w367 w370] -> w363
                    frame "S2_Ch0", Default {
                      n189 = local read "Source_2_Vcc_out"() -> (w367:refnum<k15>)
                    }
                    frame "S1_Ch2" {
                      n190 = local read "Source_1_Vcc_out"() -> (w370:refnum<k15>)
                    }
                  }
                  n191 = call <instrlib>:"niDCPower Configure Voltage Level.vi"("voltage level"=w365, "channel name"=w364, "instrument handle"=w363) -> ()  [unwired: 7 in, 2 out]
                }
                frame #1 {
                  w373 = FALSE
                  # "Отключение стабилизации"
                  n192 = while {
                    tunnel: w373 -> [_]
                    stop <- w374 stop-if-true
                    n193 = local read "NoStab"() -> (w374:bool)
                  }
                  n194 = local write "ThRes_stabil"(w373) -> ()
                }
                frame #2 {
                  # "Перестановка in0 и in1 (+ и - у Пельтье)"
                  n195 = local read "Source_2_Vcc_out"() -> (w376:refnum<k15>)
                  n196 = call <instrlib>:"niDCPower Configure Voltage Level.vi"("voltage level"=-5.0, "channel name"="2", "instrument handle"=w376) -> ()  [unwired: 7 in, 2 out]
                }
                frame #3 {
                  # "Отключение пельтье"
                  n197 = local read "Source_1_Vcc_out"() -> (w378:refnum<k15>)
                  n198 = call <instrlib>:"niDCPower Configure Voltage Level.vi"("voltage level"=0.0, "channel name"="2", "instrument handle"=w378) -> ()  [unwired: 7 in, 2 out]
                }
                frame #4 {
                  n199 = Wait (ms)(milliseconds to wait="trelax") -> ()  [unwired: 1 out]
                }
              }
              n200 = local write "Status:"("Выравнивание температуры" ("Status:")) -> ()
            }
            frame #1 {
              w389 = T4 6.5 items=["3 1/2"=3.5, "4 1/2"=4.5, "5 1/2"=5.5, "6 1/2"=6.5, "7 1/2"=7.5] ("Resolution in Digits")
              n201 = local write "Выполняется"(TRUE) -> ()
              n202 = local read "4070_address"() -> (w388:refnum<k15>)
              n203 = call-poly <instrlib>:"niDMM Config Measurement.vi"("Range"=-1.0 ("Configuration:Measurement Options:Max Frequency"), "Resolution in Digits"=w389, "Function"=niDMM_Function."2-wire Resistance" ("multimeter mode"), "instrument handle"=w388) -> ("instrument handle out"=w385:refnum<k15>)  [unwired: 6 in, 1 out]
              n204 = for {
                N: 2 -> [_]
                tunnel: w385 -> [w395]
                tunnel: [w394] -> w384
                n205 = call <instrlib>:"niDMM Read.vi"("instrument handle"=w395) -> ("instrument handle out"=w394:refnum<k15>)  [unwired: 8 in, 2 out]
              }
              n206 = for {
                N: 5 -> [_]
                tunnel: w384 -> [w397]
                tunnel: [w396] -> w387 mode=indexing
                n207 = call <instrlib>:"niDMM Read.vi"("instrument handle"=w397) -> ("Measurement"=w396:dbl)  [unwired: 8 in, 2 out]
                n208 = Wait (ms)(milliseconds to wait=u32 100) -> ()  [unwired: 1 out]
              }
              n209 = call-poly <vilib>:"Mean.vi"("X"=w387) -> ("mean"=→"Ro, Ом":dbl)  [unwired: 1 out]
              n210 = local write "Status:"("Измерение сопротивления в отсутствии тока " ("Status:")) -> ()
            }
            frame #2 {
              # "Подстройка тока\nдля пельтье"
              # "При достижении 0V поменять\nполярность, поменяв направление\nтока с помощью реле"
              n211 = Add(x="Начальное\nнапряжение TEC, В", y="Шаг напр\nдля TEC, В") -> (x+y=w399:dbl)
              n212 = for {
                N: "кол-во точек для TEC" -> [_]
                tunnel: [w429] -> w401 mode=indexing
                tunnel: [w428] -> w403 mode=indexing
                tunnel: "Шаг напр\nдля TEC, В" -> [w425]
                tunnel: [w424] -> w400 mode=indexing
                shift-right: [w427] -> _
                shift-left: w399 -> [w426]
                i -> [w423]
                # "R"
                # "I"
                # "V"
                n213 = stacked-sequence {
                  seq-local: [w431 _ _] -> [_ w460 _]
                  tunnel: [_ w461 _] -> w428
                  tunnel: [_ _ w489] -> w429
                  tunnel: [_ w460 _] -> w427
                  tunnel: w426 -> [w433 _ _]
                  tunnel: w425 -> [w432 _ _]
                  tunnel: [w430 _ _] -> w424
                  frame #0 {
                    n214 = disable-structure shown="Enabled" {
                      disable-tunnel: w433 -> [w438 w457]
                      disable-tunnel: w432 -> [w437 w458]
                      disable-tunnel: [w436 w456] -> w431
                      disable-tunnel: [w435 w455] -> w430
                      frame Disabled {
                        n215 = local read "кол-во точек для TEC"() -> (w443:i32)
                        n216 = local read "#Итерации"() -> (w440:i32)
                        n217 = Divide(x=w443, y=2) -> (x/y=w441:dbl)
                        n218 = Less?(x=w441, y=w440) -> (x < y?=w439:bool)
                        n219 = case shown="False" w439 {
                          tunnel: [0.0 -5.0] -> w444
                          tunnel: w438 -> [w447 w453]
                          tunnel: w437 -> [w446 w452]
                          tunnel: [w445 w451] -> w436
                          tunnel: [w445 w449] -> w435
                          frame False {
                            n220 = Add(x=w447, y=w446) -> (x+y=w445:dbl)
                          }
                          frame True {
                            n221 = Subtract(x=w453, y=w452) -> (x-y=w451:dbl)
                            n222 = Multiply(x=-1.0, y=w451) -> (x*y=w449:dbl)
                          }
                        }
                      }
                      frame Enabled {
                        n223 = Subtract(x=w457, y=w458) -> (x-y=w456:dbl)
                        n224 = Multiply(x=-1.0, y=w456) -> (x*y=w455:dbl)
                      }
                    }
                    n225 = Wait (ms)(milliseconds to wait=u32 100) -> ()  [unwired: 1 out]
                  }
                  frame #1 {
                    n226 = case shown="\"S1_Ch2\", Default" "TEC_Source" {
                      tunnel: [w484 w486 w488] -> w463
                      tunnel: ["2" "0" "1"] -> w462
                      frame "S1_Ch2", Default {
                        n227 = local read "Source_1_Vcc_out"() -> (w484:refnum<k15>)
                      }
                      frame "S2_Ch0" {
                        n228 = local read "Source_2_Vcc_out"() -> (w486:refnum<k15>)
                      }
                      frame "S3_Ch1" {
                        n229 = local read "Source_3_Vcc_out"() -> (w488:refnum<k15>)
                      }
                    }
                    n230 = flat-sequence {
                      tunnel: [w472] -> w467
                      tunnel: [w469] -> w466
                      tunnel: w463 -> [w471]
                      tunnel: w462 -> [w469]
                      tunnel: w460 -> [w470]
                      tunnel: w467 -> [w473]
                      tunnel: w466 -> [w474]
                      tunnel: [w474] -> w465
                      tunnel: [w473] -> w464
                      tunnel: w465 -> [w479]
                      tunnel: w464 -> [w480]
                      tunnel: [w482] -> w461
                      frame #0 {
                        n231 = call <instrlib>:"niDCPower Configure Voltage Level.vi"("voltage level"=w470, "channel name"=w469, "instrument handle"=w471) -> ("instrument handle out"=w472:refnum<k15>)  [unwired: 7 in, 1 out]
                      }
                      frame #1 {
                        n232 = Wait (ms)(milliseconds to wait=u32 100) -> ()  [unwired: 1 out]
                      }
                      frame #2 {
                        w481 = T6 0 items=["Current", "Voltage"] ("measurement type")
                        n233 = call <instrlib>:"niDCPower Measure.vi"("measurement type"=w481, "channel name"=w479, "instrument handle"=w480) -> ("measurement"=w478:dbl)  [unwired: 6 in, 2 out]
                        n234 = Multiply(x=w478, y=1000.0) -> (x*y=w476:dbl)
                        n235 = Absolute Value(x=w476) -> (abs(x)=w482:dbl)
                        "TEC_current, mA" <- w482
                      }
                    }
                  }
                  frame #2 {
                    w494 = T4 6.5 items=["3 1/2"=3.5, "4 1/2"=4.5, "5 1/2"=5.5, "6 1/2"=6.5, "7 1/2"=7.5] ("Resolution in Digits")
                    # "Снятие показаний\nТерморезистора"
                    n236 = local read "4070_address"() -> (w493:refnum<k15>)
                    n237 = call-poly <instrlib>:"niDMM Config Measurement.vi"("Range"=-1.0 ("Configuration:Measurement Options:Max Frequency"), "Resolution in Digits"=w494, "Function"=niDMM_Function."2-wire Resistance" ("multimeter mode"), "instrument handle"=w493) -> ("instrument handle out"=w492:refnum<k15>)  [unwired: 6 in, 1 out]
                    n238 = for {
                      N: 10 -> [_]
                      tunnel: w492 -> [w498]
                      tunnel: [w497] -> w491 mode=indexing
                      n239 = call <instrlib>:"niDMM Read.vi"("instrument handle"=w498) -> ("Measurement"=w497:dbl)  [unwired: 8 in, 2 out]
                      n240 = Wait (ms)(milliseconds to wait=u32 20) -> ()  [unwired: 1 out]
                    }
                    n241 = call-poly <vilib>:"Mean.vi"("X"=w491) -> ("mean"=w489:dbl)  [unwired: 1 out]
                  }
                }
                n242 = Equal?(x=0, y=w423) -> (x = y?=w421:bool)
                n243 = Select(t=u32 3000, s=w421, f="milliseconds to wait") -> (s? t:f=w420:u32)
                n244 = Wait (ms)(milliseconds to wait=w420) -> ()  [unwired: 1 out]
                "#Итерации" <- w423
              }
              n245 = local write "Status:"("Построение характеристики TEC" ("Status:")) -> ()
              n246 = flat-sequence {
                tunnel: [T1."TRes_Check(Idle)" ("Case")] -> w406
                tunnel: w403 -> [w415]
                tunnel: [TRUE] -> w404
                tunnel: w401 -> [w413]
                tunnel: w401 -> [w411]
                tunnel: w400 -> [w410]
                frame #0 {
                  # "Построение харак-ки TEC\nи опциональная запись"
                  n247 = Bundle(w415, w413) -> (→"RES(I_TEC) Graph":cluster{dbl[], dbl[]})  [unwired: 1 in]
                  n248 = Bundle(w410, w411) -> (→"RES(U_TEC) Graph":cluster{dbl[], dbl[]})  [unwired: 1 in]
                  n249 = local write "Выполняется"(FALSE) -> ()
                }
              }
            }
            frame #3 {
              n250 = disable-structure shown="Disabled" {
                frame Disabled {
                  # "Переключение в режим Вольтметра"
                  n251 = local read "4070_Rele_source"() -> (w502:enum16{"S2_Ch0", "S1_Ch2"})
                  n252 = case shown="\"S2_Ch0\", Default" w502 {
                    tunnel: [0.0 0.0] -> w505
                    tunnel: ["0" "2"] -> w504
                    tunnel: [w506 w509] -> w503
                    frame "S2_Ch0", Default {
                      n253 = local read "Source_2_Vcc_out"() -> (w506:refnum<k15>)
                    }
                    frame "S1_Ch2" {
                      n254 = local read "Source_1_Vcc_out"() -> (w509:refnum<k15>)
                    }
                  }
                  n255 = call <instrlib>:"niDCPower Configure Voltage Level.vi"("voltage level"=w505, "channel name"=w504, "instrument handle"=w503) -> ()  [unwired: 7 in, 2 out]
                }
                frame Enabled {
                }
              }
              n256 = Wait (ms)(milliseconds to wait=u32 1000) -> ()  [unwired: 1 out]
              n257 = local write "ThRes_stabil"(TRUE) -> ()
            }
          }
        }
      }
      frame "TRes_Check(Idle)" {
        w520 = T4 7.5 items=["3 1/2"=3.5, "4 1/2"=4.5, "5 1/2"=5.5, "6 1/2"=6.5, "7 1/2"=7.5] ("Resolution in Digits")
        n258 = disable-structure shown="Disabled" {
          frame Disabled {
            w549 = T4 6.5 items=["3 1/2"=3.5, "4 1/2"=4.5, "5 1/2"=5.5, "6 1/2"=6.5, "7 1/2"=7.5] ("Resolution in Digits")
            n259 = local read "4070_address"() -> (w548:refnum<k15>)
            n260 = call-poly <instrlib>:"niDMM Config Measurement.vi"("Range"=-1.0 ("Configuration:Measurement Options:Max Frequency"), "Resolution in Digits"=w549, "Function"=niDMM_Function."2-wire Resistance" ("multimeter mode"), "instrument handle"=w548) -> ("instrument handle out"=w547:refnum<k15>)  [unwired: 6 in, 1 out]
            n261 = for {
              N: 3 -> [_]
              tunnel: w547 -> [w553]
              tunnel: [w552] -> w546 mode=indexing
              n262 = call <instrlib>:"niDMM Read.vi"("instrument handle"=w553) -> ("Measurement"=w552:dbl)  [unwired: 8 in, 2 out]
              n263 = Wait (ms)(milliseconds to wait=u32 50) -> ()  [unwired: 1 out]
            }
            n264 = call-poly <vilib>:"Mean.vi"("X"=w546) -> ("mean"=→"Сопротивление терморез-ра":dbl)  [unwired: 1 out]
          }
          frame Enabled {
          }
        }
        n265 = Wait (ms)(milliseconds to wait=u32 200) -> ()  [unwired: 1 out]
        n266 = local write "Status:"("IDLE" ("Status:")) -> ()
        n267 = local read "Без Офира"() -> (w512:bool)
        n268 = local read "4071(1)_adress"() -> (w521:refnum<k15>)
        n269 = case shown="False" w512 {
          frame False {
            n270 = property on="Ophir_address" class="Ref (strict)"() -> ("Value"=w532:refnum<k7>)  [unwired: 2 in, 2 out]
            n271 = property on="hDevice" class="DigNum (strict)"() -> ("Value"=w531:i32)  [unwired: 2 in, 2 out]
            n272 = invoke class="ICoLMMeasurement" method="GetData"(reference=w532, "hDevice"=w531, "channel"=0) -> ("arrayValue"=w539:variant)  [unwired: 5 in, 7 out]
            n273 = Variant To Data(type=dbl[] [], Variant=w539) -> (data=w536:dbl[])  [unwired: 1 in, 1 out]
            n274 = Array Size(array=w536) -> (size(s)=w534:i32)
            n275 = Decrement(x=w534) -> (x-1=w533:i32)
            n276 = Index Array(array=w536, index=w533) -> (element=w535:dbl)
            n277 = Multiply(x=1000.0, y=w535) -> (x*y=→"Optical Power":dbl)
          }
          frame True {
          }
        }
        n278 = call-poly <instrlib>:"niDMM Config Measurement.vi"("Range"=-1.0 ("Configuration:Measurement Options:Max Frequency"), "Resolution in Digits"=w520, "Function"=niDMM_Function."DC Current" ("multimeter mode"), "instrument handle"=w521) -> ("instrument handle out"=w519:refnum<k15>)  [unwired: 6 in, 1 out]
        n279 = for {
          N: 5 -> [_]
          tunnel: w519 -> [w543]
          tunnel: [w541] -> w517 mode=indexing
          n280 = call <instrlib>:"niDMM Read.vi"("instrument handle"=w543) -> ("Measurement"=w541:dbl)  [unwired: 8 in, 2 out]
          n281 = Wait (ms)(milliseconds to wait=u32 50) -> ()  [unwired: 1 out]
        }
        n282 = call-poly <vilib>:"Mean.vi"("X"=w517) -> ("mean"=w516:dbl)  [unwired: 1 out]
        n283 = Absolute Value(x=w516) -> (abs(x)=w515:dbl)
        n284 = Multiply(x=w515, y=1000000.0) -> (x*y=w513:dbl)
        n285 = local write "I_pd, uA"(w513) -> ()
        n286 = Select(t=T1."Quit" ("Case"), s="stop", f=T1."TRes_Check(Idle)" ("Case")) -> (s? t:f=w527:T1)
      }
      frame "Characteristics" {
        n287 = flat-sequence {
          tunnel: [w575] -> w565
          tunnel: [w579] -> w563
          tunnel: [w578] -> w561
          tunnel: [w577] -> w559
          tunnel: [w574] -> w557
          tunnel: [w572] -> w555
          tunnel: w565 -> [w818]
          tunnel: [w818] -> w564
          tunnel: w563 -> [w803]
          tunnel: [w803] -> w562
          tunnel: w561 -> [w820]
          tunnel: [w820] -> w560
          tunnel: w559 -> [w804]
          tunnel: [w804] -> w558
          tunnel: w557 -> [w819]
          tunnel: [w819] -> w556
          tunnel: w555 -> [w794]
          tunnel: [T1."TRes_Check(Idle)" ("Case")] -> w567
          tunnel: w564 -> [w821]
          tunnel: w562 -> [w841]
          tunnel: w560 -> [w840]
          tunnel: w558 -> [w838]
          tunnel: w556 -> [w835]
          frame #0 {
            n288 = local read "Отладка(F)/\n/Рабочий(T)"() -> (w568:bool)
            n289 = case shown="True" w568 {
              frame False {
              }
              frame True {
                n290 = while {
                  stop <- w570 stop-if-true
                  n291 = call "Save_dialogue_dose.vi"() -> ("output 1"=w569:dbl)  [unwired: 11 in]
                  n292 = Not Equal To 0?(x=w569) -> (x != 0?=w570:bool)
                  n293 = property on="Dose" class="DigNum (strict)"("Value"=w569) -> ()  [unwired: 2 in, 2 out]
                }
              }
            }
          }
          frame #1 {
            # "Хар-ки:\nI_LD (V);\nOphir(I_LD);\nI_PD(I_LD);\nRcheck(I_LD)"
            n294 = Subtract(x="Начальный ток, мА", y="Шаг, мА") -> (x-y=w580:dbl)
            n295 = for {
              N: "Кол-во точек" -> [_]
              shift-right: [w591] -> _
              shift-left: w580 -> [w593]
              tunnel: [w591] -> w575 mode=indexing
              tunnel: [w590] -> w579 mode=indexing
              tunnel: [w589] -> w578 mode=indexing
              tunnel: [w588] -> w577 mode=indexing
              tunnel: [w586] -> w574 mode=indexing
              tunnel: [w584] -> w572
              shift-right: [w582] -> _
              shift-left: "Start voltage_LD" -> [w583]
              i -> [w587]
              # "ExtPD"
              # "FV"
              # "I_PD"
              # "I_LD"
              # "Ophir"
              n296 = property on="Шаг, мА" class="DigNum (strict)"() -> ("Value"=w585:dbl)  [unwired: 2 in, 2 out]
              n297 = Add(x=w593, y=w585) -> (x+y=w592:dbl)
              n298 = stacked-sequence {
                tunnel: w592 -> [_ w615 _ _ _ _ _ _ _]
                tunnel: [_ w610 _ _ _ _ _ _ _] -> w591
                tunnel: [_ _ _ _ _ w678 _ _ _] -> w590
                tunnel: [_ _ _ _ _ _ w696 _ _] -> w589
                tunnel: [_ _ _ _ w668 _ _ _ _] -> w588
                tunnel: w587 -> [_ _ _ _ _ _ _ _ w733]
                tunnel: [_ _ _ _ _ _ _ w709 _] -> w586
                tunnel: [_ _ _ _ _ _ _ _ w732] -> w584
                tunnel: w583 -> [_ w607 _ _ _ _ _ _ _]
                tunnel: [_ w606 _ _ _ _ _ _ _] -> w582
                frame #0 {
                  n299 = disable-structure shown="Disabled" {
                    frame Disabled {
                      n300 = stacked-sequence {
                        frame #0 {
                          w594 = FALSE
                          # "Отключение стабилизации"
                          n301 = while {
                            tunnel: w594 -> [_]
                            stop <- w595 stop-if-true
                            n302 = local read "NoStab"() -> (w595:bool)
                          }
                          n303 = local write "ThRes_stabil"(w594) -> ()
                        }
                        frame #1 {
                          # "Переключение в режим Вольтметра"
                          n304 = local read "4070_Rele_source"() -> (w596:enum16{"S2_Ch0", "S1_Ch2"})
                          n305 = case shown="\"S2_Ch0\", Default" w596 {
                            tunnel: [0.0 0.0] -> w599
                            tunnel: ["0" "2"] -> w598
                            tunnel: [w600 w603] -> w597
                            frame "S2_Ch0", Default {
                              n306 = local read "Source_2_Vcc_out"() -> (w600:refnum<k15>)
                            }
                            frame "S1_Ch2" {
                              n307 = local read "Source_1_Vcc_out"() -> (w603:refnum<k15>)
                            }
                          }
                          n308 = call <instrlib>:"niDCPower Configure Voltage Level.vi"("voltage level"=w599, "channel name"=w598, "instrument handle"=w597) -> ()  [unwired: 7 in, 2 out]
                        }
                      }
                    }
                    frame Enabled {
                    }
                  }
                }
                frame #1 {
                  # "Подстройка тока\nлазерного диода"
                  n309 = local read "Source_1_Vcc_out"() -> (w616:refnum<k15>)
                  n310 = disable-structure shown="Enabled" {
                    disable-tunnel: "the lower limit for the voltage_LD" -> [w632 w638]
                    disable-tunnel: w607 -> [w631 w639]
                    disable-tunnel: "the upper limit for the voltage_LD" -> [w630 w640]
                    disable-tunnel: w616 -> [w629 w637]
                    disable-tunnel: w615 -> [w628 w636]
                    disable-tunnel: "Res_LD" -> [w627 w635]
                    disable-tunnel: "0" -> [w626 w633]
                    disable-tunnel: "accuracy_LD" -> [w625 w643]
                    disable-tunnel: [w624 w642] -> w606
                    disable-tunnel: [w622 w641] -> w611
                    disable-tunnel: [w621 w634] -> w610
                    frame Disabled {
                      n311 = local read "4070_address"() -> (w623:refnum<k15>)
                      n312 = call "Set input current_ChAmmeter.vi"("the lower limit for the voltage"=w632, "accuracy (input)"=w625, "4070_address"=w623, "Start voltage"=w631, "the upper limit for the voltage"=w630, "instrument handle"=w629, "the optimum current(input)"=w628, "res(input)"=w627, "channel name"=w626) -> ("accommodated voltage (out)"=w624:dbl, "current value, mA"=w621:dbl, "the voltage drop across the resistor"=w622:dbl)  [unwired: 3 in, 1 out]
                    }
                    frame Enabled {
                      n313 = call "Set input current_ChSource.vi"("channel name"=w633, "res(input)"=w635, "the optimum current(input)"=w636, "accuracy (input)"=w643, "instrument handle"=w637, "the upper limit for the voltage"=w640, "Start voltage"=w639, "the lower limit for the voltage"=w638) -> ("current value, mA"=w634:dbl, "the voltage drop across the resistor"=w641:dbl, "accommodated voltage (out)"=w642:dbl)  [unwired: 1 out]
                    }
                  }
                  "Подстроенный ток, mA" <- w610
                  "accommodated voltage (out)" <- w606
                  "Volt_onRes" <- w611
                  n314 = local write "Status:"("Подстройка тока LD" ("Status:")) -> ()
                  n315 = Wait (ms)(milliseconds to wait=u32 100) -> ()  [unwired: 1 out]
                  n316 = Greater Or Equal?(x=w610, y=49.5) -> (x >= y?=→"Boolean":bool)
                }
                frame #2 {
                  # "and stab"
                  # "Resistance check"
                  n317 = flat-sequence {
                    frame #0 {
                      n318 = disable-structure shown="Disabled" {
                        frame Disabled {
                          # "Режим Омметра"
                          n319 = case shown="\"S2_Ch0\", Default" "4070_Rele_source" {
                            tunnel: [5.0 -5.0] -> w647
                            tunnel: ["0" "2"] -> w646
                            tunnel: [w649 w652] -> w645
                            frame "S2_Ch0", Default {
                              n320 = local read "Source_2_Vcc_out"() -> (w649:refnum<k15>)
                            }
                            frame "S1_Ch2" {
                              n321 = local read "Source_1_Vcc_out"() -> (w652:refnum<k15>)
                            }
                          }
                          n322 = call <instrlib>:"niDCPower Configure Voltage Level.vi"("voltage level"=w647, "channel name"=w646, "instrument handle"=w645) -> ()  [unwired: 7 in, 2 out]
                        }
                        frame Enabled {
                        }
                      }
                    }
                    frame #1 {
                      n323 = Wait (ms)(milliseconds to wait=u32 1000) -> ()  [unwired: 1 out]
                      "Num_hits" <- u64 0 ("Num_hits")
                    }
                    frame #2 {
                      n324 = local write "ThRes_stabil"(TRUE) -> ()
                    }
                    frame #3 {
                      n325 = local write "Count_hits?"(TRUE ("Acq_allow?")) -> ()
                      n326 = Wait (ms)(milliseconds to wait="tstab между точками, мс") -> ()  [unwired: 1 out]
                    }
                  }
                  n327 = local write "Status:"("Проверка и стабилизация сопротивления" ("Status:")) -> ()
                }
                frame #3 {
                  n328 = while {
                    tunnel: [u64 0] -> w661
                    tunnel: [FALSE ("Acq_allow?")] -> w660
                    stop <- w664 stop-if-true
                    n329 = local read "Num_hits"() -> (w666:u64)
                    n330 = Greater Or Equal?(x=w666, y="Num_hits_req") -> (x >= y?=w664:bool)
                  }
                  n331 = local write "Count_hits?"(w660) -> ()
                  n332 = local write "Num_hits"(w661) -> ()
                }
                frame #4 {
                  # "Forward\nVoltage\nmeasurement"
                  n333 = local read "Source_1_Vcc_out"() -> (w674:refnum<k15>)
                  n334 = local read "Volt_onRes"() -> (w667:dbl)
                  n335 = call <instrlib>:"niDCPower Measure Multiple.vi"("channel name"="0", "instrument handle"=w674) -> ("voltage measurements"=w672:dbl[])  [unwired: 6 in, 3 out]
                  n336 = Index Array(array=w672) -> (element=w670:dbl)  [unwired: 1 in]
                  n337 = Absolute Value(x=w667) -> (abs(x)=w669:dbl)
                  n338 = Absolute Value(x=w670) -> (abs(x)=w671:dbl)
                  n339 = Subtract(x=w671, y=w669) -> (x-y=w668:dbl)
                  "Forward Voltage, V" <- w668
                  n340 = local write "Status:"("Измерение прямого напряжения" ("Status:")) -> ()
                  n341 = Wait (ms)(milliseconds to wait=u32 100) -> ()  [unwired: 1 out]
                }
                frame #5 {
                  n342 = local read "Без Офира"() -> (w677:bool)
                  n343 = case shown="True" w677 {
                    tunnel: [w679 1.0] -> w678
                    frame False {
                      # "Ophir\nmeasurement"
                      n344 = property on="Ophir_address" class="Ref (strict)"() -> ("Value"=w681:refnum<k7>)  [unwired: 2 in, 2 out]
                      n345 = property on="hDevice" class="DigNum (strict)"() -> ("Value"=w680:i32)  [unwired: 2 in, 2 out]
                      n346 = invoke class="ICoLMMeasurement" method="GetData"(reference=w681, "hDevice"=w680, "channel"=0) -> ("arrayValue"=w688:variant)  [unwired: 5 in, 7 out]
                      n347 = local write "Status:"("Измерен. оптич. мощности" ("Status:")) -> ()
                      n348 = Variant To Data(type=dbl[] [], Variant=w688) -> (data=w685:dbl[])  [unwired: 1 in, 1 out]
                      n349 = Wait (ms)(milliseconds to wait=u32 200) -> ()  [unwired: 1 out]
                      n350 = Array Size(array=w685) -> (size(s)=w683:i32)
                      n351 = Decrement(x=w683) -> (x-1=w682:i32)
                      n352 = Index Array(array=w685, index=w682) -> (element=w684:dbl)
                      n353 = Multiply(x=1000.0, y=w684) -> (x*y=w679:dbl)
                      "Ophir, mW" <- w679
                      n354 = local write "Optical Power"(w679) -> ()
                    }
                    frame True {
                    }
                  }
                }
                frame #6 {
                  w699 = T4 7.5 items=["3 1/2"=3.5, "4 1/2"=4.5, "5 1/2"=5.5, "6 1/2"=6.5, "7 1/2"=7.5] ("Resolution in Digits")
                  # "Inside I_PD\nmeasurements"
                  n355 = local read "4071(1)_adress"() -> (w700:refnum<k15>)
                  n356 = call-poly <instrlib>:"niDMM Config Measurement.vi"("Range"=-1.0 ("Configuration:Measurement Options:Max Frequency"), "Resolution in Digits"=w699, "Function"=niDMM_Function."DC Current" ("multimeter mode"), "instrument handle"=w700) -> ("instrument handle out"=w698:refnum<k15>)  [unwired: 6 in, 1 out]
                  n357 = for {
                    N: 5 -> [_]
                    tunnel: w698 -> [w707]
                    tunnel: [w704] -> w693 mode=indexing
                    n358 = call <instrlib>:"niDMM Read.vi"("instrument handle"=w707) -> ("Measurement"=w705:dbl)  [unwired: 8 in, 2 out]
                    n359 = Absolute Value(x=w705) -> (abs(x)=w704:dbl)
                    n360 = Wait (ms)(milliseconds to wait=u32 50) -> ()  [unwired: 1 out]
                  }
                  n361 = local write "Status:"("I_PD встроенного фотодиода" ("Status:")) -> ()
                  n362 = call-poly <vilib>:"Mean.vi"("X"=w693) -> ("mean"=w694:dbl)  [unwired: 1 out]
                  n363 = Multiply(x=w694, y=1000000.0) -> (x*y=w696:dbl)
                  "I_pd, uA" <- w696
                }
                frame #7 {
                  # "EXTERNAL I_PD\nmeasurements"
                  n364 = disable-structure shown="Enabled" {
                    disable-tunnel: [w712 w727] -> w709
                    disable-tunnel: [_ w727] -> w708
                    frame Disabled {
                      w719 = T4 6.5 items=["3 1/2"=3.5, "4 1/2"=4.5, "5 1/2"=5.5, "6 1/2"=6.5, "7 1/2"=7.5] ("Resolution in Digits")
                      n365 = local read "4071(2)_adress"() -> (w720:refnum<k15>)
                      n366 = call-poly <instrlib>:"niDMM Config Measurement.vi"("Range"=-1.0 ("Configuration:Measurement Options:Max Frequency"), "Resolution in Digits"=w719, "Function"=niDMM_Function."DC Current" ("multimeter mode"), "instrument handle"=w720) -> ("instrument handle out"=w718:refnum<k15>)  [unwired: 6 in, 1 out]
                      n367 = for {
                        N: 5 -> [_]
                        tunnel: w718 -> [w725]
                        tunnel: [w723] -> w716 mode=indexing
                        n368 = call <instrlib>:"niDMM Read.vi"("instrument handle"=w725) -> ("Measurement"=w723:dbl)  [unwired: 8 in, 2 out]
                        n369 = Wait (ms)(milliseconds to wait=u32 50) -> ()  [unwired: 1 out]
                      }
                      n370 = call-poly <vilib>:"Mean.vi"("X"=w716) -> ("mean"=w715:dbl)  [unwired: 1 out]
                      n371 = Absolute Value(x=w715) -> (abs(x)=w714:dbl)
                      n372 = Multiply(x=w714, y=1000.0) -> (x*y=w712:dbl)
                    }
                    frame Enabled {
                      n373 = local read "Source_2_Vcc_out"() -> (w731:refnum<k15>)
                      n374 = call <instrlib>:"niDCPower Measure Multiple.vi"("channel name"="1", "instrument handle"=w731) -> ("current measurements"=w729:dbl[])  [unwired: 6 in, 3 out]
                      n375 = Index Array(array=w729) -> (element=w726:dbl)  [unwired: 1 in]
                      n376 = Multiply(x=w726, y=1000.0) -> (x*y=w727:dbl)
                    }
                  }
                  "IPD(ext), mA" <- w708
                  n377 = local write "Status:"("I_PD внешнего фотодиода" ("Status:")) -> ()
                  n378 = Wait (ms)(milliseconds to wait=u32 200) -> ()  [unwired: 1 out]
                }
                frame #8 {
                  n379 = local read "Отладка(F)/\n/Рабочий(T)"() -> (w734:bool)
                  n380 = case shown="True" w734 {
                    tunnel: w733 -> [_ w753]
                    tunnel: [_ w735] -> w732
                    frame False {
                    }
                    frame True {
                      w743 = i16 3 ("width (-)")
                      w744 = i16 3 ("width (-)")
                      w746 = i16 3 ("width (-)")
                      w749 = i16 3 ("width (-)")
                      w752 = i16 3 ("width (-)")
                      # "Внешний ФД"
                      # "Офир"
                      n381 = local read "IPD(ext), mA"() -> (w737:dbl)
                      n382 = local read "Ophir, mW"() -> (w736:dbl)
                      n383 = local read "Forward Voltage, V"() -> (w748:dbl)
                      n384 = local read "Подстроенный ток, mA"() -> (w751:dbl)
                      n385 = local read "I_pd, uA"() -> (w745:dbl)
                      n386 = Equal To 0?(x=w753) -> (x = 0?=w741:bool)
                      n387 = Number To Fractional String(number=w751, width (-)=w752, precision (6)=w752) -> (F-format string=w750:string)  [unwired: 1 in]
                      n388 = Number To Fractional String(number=w748, width (-)=w749, precision (6)=w749) -> (F-format string=w747:string)  [unwired: 1 in]
                      n389 = Number To Fractional String(number=w737, width (-)=w746, precision (6)=w746) -> (F-format string=w738:string)  [unwired: 1 in]
                      n390 = Number To Fractional String(number=w745, width (-)=w744, precision (6)=w744) -> (F-format string=w739:string)  [unwired: 1 in]
                      n391 = Number To Fractional String(number=w736, width (-)=w743, precision (6)=w743) -> (F-format string=w740:string)  [unwired: 1 in]
                      n392 = case shown="True" w741 {
                        tunnel: ["" ("date/time string") w759] -> w735
                        tunnel: ["" w756] -> w742
                        frame False {
                        }
                        frame True {
                          w758 = i16 0 ("width (-)")
                          n393 = Get Date/Time In Seconds() -> (seconds since 1Jan1904=w761:timestamp)
                          n394 = Format Date/Time String(time format string (%c)="%d  %H:%M:%S", seconds (now)=w761) -> (date/time string=w759:string)  [unwired: 1 in]
                          n395 = Number To Fractional String(number="Dose", width (-)=w758, precision (6)=w758) -> (F-format string=w756:string)  [unwired: 1 in]
                        }
                      }
                      n396 = stacked-sequence {
                        tunnel: w735 -> [w769 w777 w785 _ w793]
                        tunnel: w742 -> [w767 w774 w782 _ w791]
                        tunnel: w750 -> [w765 w773 w781 _ w787]
                        tunnel: w747 -> [w763 _ _ _ _]
                        tunnel: w740 -> [_ w772 _ _ _]
                        tunnel: w739 -> [_ _ w779 _ _]
                        tunnel: w738 -> [_ _ _ _ w789]
                        frame #0 {
                          w764 = "\t"
                          n397 = local read "V2(Ild)_Log_address"() -> (w768:refnum<file>)
                          n398 = Format Into String(initial string=w768, w769, w764, "", w764, w767, w764, w765, w764, w763, "\r\n") -> ()  [unwired: 2 in, 2 out]
                        }
                        frame #1 {
                          w771 = "\t"
                          n399 = local read "Op(Ild)_Log_address"() -> (w776:refnum<file>)
                          n400 = Format Into String(initial string=w776, w777, w771, "", w771, w774, w771, w773, w771, w772, "\r\n") -> ()  [unwired: 2 in, 2 out]
                        }
                        frame #2 {
                          w780 = "\t"
                          n401 = local read "Ipd(Ild)_Monitor_Log_address"() -> (w784:refnum<file>)
                          n402 = Format Into String(initial string=w784, w785, w780, "", w780, w782, w780, w781, w780, w779, "\r\n") -> ()  [unwired: 2 in, 2 out]
                        }
                        frame #3 {
                        }
                        frame #4 {
                          w788 = "\t"
                          n403 = local read "Ipd(Ild)_External_Log_address"() -> (w792:refnum<file>)
                          n404 = Format Into String(initial string=w792, w793, w788, "", w788, w791, w788, w787, w788, w789, "\r\n") -> ()  [unwired: 2 in, 2 out]
                        }
                      }
                    }
                  }
                }
              }
            }
          }
          frame #2 {
            w800 = i16 3 ("width (-)")
            w806 = i16 3 ("width (-)")
            w808 = i16 3 ("width (-)")
            w811 = i16 3 ("width (-)")
            w813 = "" ("input 1")
            w798 = "\t"
            w816 = i16 3 ("width (-)")
            # "Рабочее напряжение"
            n405 = local read "Подстроенный ток, mA"() -> (w810:dbl)
            n406 = local read "Ophir, mW"() -> (w805:dbl)
            n407 = call "Find_ThresholdOphir_F4.vi"("Threshold Ophir"=5.0, "Current array"=w804, "Ophir array"=w803) -> ("Threshold Current"=w801:dbl)  [unwired: 8 in]
            n408 = call "Find_ThresholdOphir_F4.vi"("Threshold Ophir"=1.0, "Current array"=w818, "Ophir array"=w803) -> ("Threshold Current"=w815:dbl)  [unwired: 8 in]
            "Пороговый ток" <- w815
            n409 = local read "I_pd, uA"() -> (w799:dbl)
            n410 = Number To Fractional String(number=w801, width (-)=w808, precision (6)=w808) -> (F-format string=w807:string)  [unwired: 1 in]
            n411 = Number To Fractional String(number=w815, width (-)=w816, precision (6)=w816) -> (F-format string=w812:string)  [unwired: 1 in]
            n412 = Number To Fractional String(number=w799, width (-)=w800, precision (6)=w800) -> (F-format string=w796:string)  [unwired: 1 in]
            n413 = Number To Fractional String(number=w805, width (-)=w806, precision (6)=w806) -> (F-format string=w795:string)  [unwired: 1 in]
            n414 = Number To Fractional String(number=w810, width (-)=w811, precision (6)=w811) -> (F-format string=w809:string)  [unwired: 1 in]
            n415 = local read "Param_Log_address"() -> (w814:refnum<file>)
            n416 = Format Into String(initial string=w814, w794, w798, w813, w798, w813, w798, w812, w798, w809, w798, w807, w798, w796, w798, w795, "\r\n") -> ()  [unwired: 2 in, 2 out]
          }
          frame #3 {
            n417 = property on="Boolean" class="Bool (strict)"() -> ("Value"=w830:bool)  [unwired: 2 in, 2 out]
            n418 = And(x=w830, y="Оставить в раб.\nрежиме") -> (x .and. y?=w831:bool)
            n419 = local read "Source_1_Vcc_out"() -> (w833:refnum<k15>)
            n420 = local read "Подстроенное напряжение\nстабилизации"() -> (w827:dbl)
            n421 = case shown="True" w831 {
              tunnel: [0.0 ("voltage level") w846] -> w832
              frame False {
              }
              frame True {
                n422 = local read "accommodated voltage (out)"() -> (w846:dbl)
              }
            }
            n423 = local read "Source_1_Vcc_out"() -> (w826:refnum<k15>)
            n424 = Bundle(w821, w841) -> (→"OP(I_LD) Graph":cluster{dbl[], dbl[]})  [unwired: 1 in]
            n425 = Bundle(w821, w840) -> (→"I_PD(I_LD) Graph":cluster{dbl[], dbl[]})  [unwired: 1 in]
            n426 = Bundle(w821, w838) -> (→"V2(I_LD) Graph":cluster{dbl[], dbl[]})  [unwired: 1 in]
            n427 = Bundle(w821, w835) -> (→"I_PD_Ext(I_LD) Graph":cluster{dbl[], dbl[]})  [unwired: 1 in]
            n428 = Add(x=w827, y=0.2) -> (x+y=w822:dbl)
            n429 = local write "Выполняется"(FALSE) -> ()
            n430 = Multiply(x=w822, y=-1.0) -> (x*y=w823:dbl)
            n431 = call <instrlib>:"niDCPower Configure Voltage Level.vi"("voltage level"=w823, "channel name"="2", "instrument handle"=w826) -> ()  [unwired: 7 in, 2 out]
            n432 = call <instrlib>:"niDCPower Configure Voltage Level.vi"("voltage level"=w832, "channel name"="0", "instrument handle"=w833) -> ()  [unwired: 7 in, 2 out]
          }
        }
        n433 = local write "Boolean 2"(FALSE) -> ()
      }
      frame "Bias" {
        n434 = local write "Boolean 2"(FALSE) -> ()
        n435 = stacked-sequence {
          tunnel: [_ _ _ T1."TRes_Check(Idle)" ("Case")] -> w848
          frame #0 {
            n436 = disable-structure shown="Disabled" {
              frame Disabled {
                w850 = FALSE
                n437 = while {
                  tunnel: w850 -> [_]
                  stop <- w851 stop-if-true
                  n438 = local read "NoStab"() -> (w851:bool)
                }
                n439 = local write "ThRes_stabil"(w850) -> ()
              }
              frame Enabled {
              }
            }
            n440 = local write "Num_hits"(0) -> ()
          }
          frame #1 {
            n441 = disable-structure shown="Disabled" {
              frame Disabled {
                # "Переключение в режим Вольтметра"
                n442 = local read "4070_Rele_source"() -> (w852:enum16{"S2_Ch0", "S1_Ch2"})
                n443 = case shown="\"S2_Ch0\", Default" w852 {
                  tunnel: [0.0 0.0] -> w855
                  tunnel: ["0" "2"] -> w854
                  tunnel: [w856 w859] -> w853
                  frame "S2_Ch0", Default {
                    n444 = local read "Source_2_Vcc_out"() -> (w856:refnum<k15>)
                  }
                  frame "S1_Ch2" {
                    n445 = local read "Source_1_Vcc_out"() -> (w859:refnum<k15>)
                  }
                }
                n446 = call <instrlib>:"niDCPower Configure Voltage Level.vi"("voltage level"=w855, "channel name"=w854, "instrument handle"=w853) -> ()  [unwired: 7 in, 2 out]
              }
              frame Enabled {
              }
            }
          }
          frame #2 {
            n447 = local read "the upper limit for the voltage_LD"() -> (w876:dbl)
            n448 = local read "the lower limit for the voltage_LD"() -> (w878:dbl)
            n449 = local read "Source_1_Vcc_out"() -> (w875:refnum<k15>)
            n450 = local read "Start voltage_LD"() -> (w877:dbl)
            n451 = local read "accuracy_LD"() -> (w872:dbl)
            n452 = local read "Res_LD"() -> (w874:dbl)
            n453 = disable-structure shown="Enabled" {
              disable-tunnel: "Desirable Operating current, mA" -> [w891 w897]
              disable-tunnel: [w890 w898] -> w879
              disable-tunnel: w878 -> [w889 w901]
              disable-tunnel: w877 -> [w888 w892]
              disable-tunnel: w876 -> [w887 w893]
              disable-tunnel: w875 -> [w886 w894]
              disable-tunnel: w874 -> [w885 w896]
              disable-tunnel: "0" ("channel name") -> [w884 w895]
              disable-tunnel: w872 -> [w883 w900]
              disable-tunnel: [w882 w899] -> w871
              frame Disabled {
                n454 = local read "4070_address"() -> (w881:refnum<k15>)
                n455 = call "Set input current_ChAmmeter.vi"("the lower limit for the voltage"=w889, "accuracy (input)"=w883, "4070_address"=w881, "Start voltage"=w888, "the upper limit for the voltage"=w887, "instrument handle"=w886, "the optimum current(input)"=w891, "res(input)"=w885, "channel name"=w884) -> ("accommodated voltage (out)"=w882:dbl, "current value, mA"=w890:dbl)  [unwired: 3 in, 2 out]
              }
              frame Enabled {
                n456 = call "Set input current_ChSource.vi"("channel name"=w895, "res(input)"=w896, "the optimum current(input)"=w897, "accuracy (input)"=w900, "instrument handle"=w894, "the upper limit for the voltage"=w893, "Start voltage"=w892, "the lower limit for the voltage"=w901) -> ("current value, mA"=w898:dbl, "accommodated voltage (out)"=w899:dbl)  [unwired: 2 out]
              }
            }
            "Operating Current, mA" <- w879
            n457 = local read "+ V TEC для новой точки"() -> (w866:dbl)
            n458 = local read "Подстроенное напряжение\nстабилизации"() -> (w864:dbl)
            n459 = local read "Source_1_Vcc_out"() -> (w870:refnum<k15>)
            n460 = local write "accommodated voltage (out)"(w871) -> ()
            n461 = Multiply(x=w866, y=2.0) -> (x*y=w863:dbl)
            n462 = Add(x=w863, y=w864) -> (x+y=w862:dbl)
            n463 = Multiply(x=w862, y=-1.0) -> (x*y=w867:dbl)
            n464 = call <instrlib>:"niDCPower Configure Voltage Level.vi"("voltage level"=w867, "channel name"="2", "instrument handle"=w870) -> ()  [unwired: 7 in, 2 out]
          }
          frame #3 {
            n465 = disable-structure shown="Enabled" {
              frame Disabled {
                # "Переключение в режим Омметра"
                n466 = local read "4070_Rele_source"() -> (w908:enum16{"S2_Ch0", "S1_Ch2"})
                n467 = case shown="\"S2_Ch0\", Default" w908 {
                  tunnel: [5.0 -5.0] -> w907
                  tunnel: ["0" "2"] -> w906
                  tunnel: [w909 w912] -> w905
                  frame "S2_Ch0", Default {
                    n468 = local read "Source_2_Vcc_out"() -> (w909:refnum<k15>)
                  }
                  frame "S1_Ch2" {
                    n469 = local read "Source_1_Vcc_out"() -> (w912:refnum<k15>)
                  }
                }
                n470 = call <instrlib>:"niDCPower Configure Voltage Level.vi"("voltage level"=w907, "channel name"=w906, "instrument handle"=w905) -> ()  [unwired: 7 in, 2 out]
              }
              frame Enabled {
              }
            }
            n471 = local write "Выполняется"(FALSE) -> ()
            n472 = local write "ThRes_stabil"(TRUE) -> ()
          }
        }
      }
      frame "Quit" {
        w916 = FALSE
        n473 = local write "Status:"("Выход" ("Status:")) -> ()
        n474 = local write "Num_hits"(u64 0 ("Num_hits")) -> ()
        n475 = local write "stop"(w916) -> ()
        n476 = local write "Power Enable"(w916) -> ()
        n477 = local write "Прервать"(w916) -> ()
        n478 = local write "Count_hits?"(w916) -> ()
      }
    }
  }
  n479 = while {
    tunnel: w6 -> [w921]
    stop <- FALSE stop-if-true
    n480 = event shown="[0] \"stop\": Value Change" {
      selector: _ -> [_ _ _ _]
      dyn-events: _ -> [_ _ _ _]
      timeout: _ -> [_ _ _ _]
      tunnel: w921 -> [_ _ _ _]
      event "stop": Value Change {
        # "Работает, зараза, через раз"
        n481 = event-data() -> ()  [unwired: 1 in, 6 out]
        n482 = flat-sequence {
          frame #0 {
            n483 = local write "Case"(T1."Quit" ("Case")) -> ()
          }
          frame #1 {
            n484 = local write "stop"(FALSE) -> ()
            "Прервать" <- TRUE
          }
        }
      }
      event "Раб. режим LD": Value Change {
        n485 = event-data() -> ()  [unwired: 1 in, 6 out]
        n486 = flat-sequence {
          frame #0 {
            n487 = local write "Раб. режим LD"(FALSE) -> ()
            n488 = local write "Case"(T1."Bias" ("Case")) -> ()
          }
          frame #1 {
            n489 = local write "Выполняется"(TRUE) -> ()
          }
        }
      }
      event "Хар-ка TEC": Value Change {
        n490 = event-data() -> ()  [unwired: 1 in, 6 out]
        n491 = flat-sequence {
          frame #0 {
            n492 = local write "Хар-ка TEC"(FALSE) -> ()
            n493 = local write "Case"(T1."TEC_Chars" ("Case")) -> ()
          }
          frame #1 {
            n494 = local write "Выполняется"(TRUE) -> ()
          }
        }
      }
      event "Хар-ки от I_LD": Value Change {
        n495 = event-data() -> ()  [unwired: 1 in, 6 out]
        n496 = flat-sequence {
          frame #0 {
            n497 = local write "Хар-ки от I_LD"(FALSE) -> ()
            n498 = local write "Case"(T1."Characteristics" ("Case")) -> ()
          }
          frame #1 {
            n499 = local write "Выполняется"(TRUE) -> ()
          }
        }
      }
    }
  }
  n500 = while {
    tunnel: w1 -> [w935]
    tunnel: w4 -> [w936]
    stop <- FALSE stop-if-true
    w938 = T1."Initialization"  # Case
    n501 = disable-structure shown="Enabled" {
      frame Disabled {
        n502 = local read "Выполняется"() -> (w940:bool)
        n503 = Compound Arithmetic op=OR(w940) -> ()  [unwired: 1 in, 1 out]
      }
      frame Enabled {
      }
    }
    n504 = local read "Case"() -> (w937:T1)
    n505 = Equal?(x=w937, y=w938) -> (x = y?=w934:bool)
    n506 = case shown="False" w934 {
      tunnel: w936 -> [w942 _]
      tunnel: w935 -> [w941 _]
      frame False {
        n507 = stacked-sequence {
          tunnel: w942 -> [w944 w982 _]
          tunnel: w941 -> [w943 w981 _]
          frame #0 {
            n508 = disable-structure shown="Enabled" {
              disable-tunnel: w944 -> [w947 _]
              disable-tunnel: w943 -> [w946 _]
              frame Enabled {
                n509 = local read "Power Enable"() -> (w945:bool)
                n510 = call <instrlib>:"niDCPower Configure Output Enabled.vi"("output enabled"=w945, "channel name"="0,1,2", "instrument handle"=w947) -> ()  [unwired: 7 in, 2 out]
                n511 = call <instrlib>:"niDCPower Configure Output Enabled.vi"("output enabled"=w945, "channel name"="0,1,2", "instrument handle"=w946) -> ()  [unwired: 7 in, 2 out]
              }
              frame Disabled {
              }
            }
          }
          frame #1 {
            w961 = "1"
            w965 = 1000.0 ("y")
            w972 = "0" ("channel name")
            n512 = Divide(x="Предел тока ТЕС, мА", y=1000.0) -> (x/y=w975:dbl)
            n513 = call <instrlib>:"niDCPower Configure Current Limit.vi"("current limit"=w975, "channel name"="2", "instrument handle"=w982) -> ("instrument handle out"=w954:refnum<k15>)  [unwired: 7 in, 1 out]
            n514 = call <instrlib>:"niDCPower Configure Current Limit.vi"("current limit"=w975, "channel name"="0", "instrument handle"=w981) -> ("instrument handle out"=w968:refnum<k15>)  [unwired: 7 in, 1 out]
            n515 = Divide(x="Предел тока LD, мА", y=w965) -> (x/y=w976:dbl)
            n516 = Divide(x="Предел тока PDext, мА", y=w965) -> (x/y=w967:dbl)
            n517 = call <instrlib>:"niDCPower Configure Current Limit.vi"("current limit"=w967, "channel name"=w961, "instrument handle"=w968) -> ("instrument handle out"=w960:refnum<k15>)  [unwired: 7 in, 1 out]
            n518 = call <instrlib>:"niDCPower Measure Multiple.vi"("channel name"="2", "instrument handle"=w954) -> ("current measurements"=w957:dbl[])  [unwired: 6 in, 3 out]
            n519 = call <instrlib>:"niDCPower Configure Current Limit.vi"("current limit"=w976, "channel name"=w972, "instrument handle"=w954) -> ("instrument handle out"=w973:refnum<k15>)  [unwired: 7 in, 1 out]
            n520 = call <instrlib>:"niDCPower Measure Multiple.vi"("channel name"=w961, "instrument handle"=w960) -> ("current measurements"=w962:dbl[])  [unwired: 6 in, 3 out]
            n521 = Index Array(array=w957) -> (element=w956:dbl)  [unwired: 1 in]
            n522 = call <instrlib>:"niDCPower Measure Multiple.vi"("channel name"=w972, "instrument handle"=w973) -> ("current measurements"=w971:dbl[])  [unwired: 6 in, 3 out]
            n523 = Multiply(x=w956, y=1000.0) -> (x*y=w958:dbl)
            n524 = Index Array(array=w962) -> (element=w963:dbl)  [unwired: 1 in]
            n525 = Absolute Value(x=w958) -> (abs(x)=w952:dbl)
            n526 = Index Array(array=w971) -> (element=w970:dbl)  [unwired: 1 in]
            n527 = Multiply(x=w963, y=1000.0) -> (x*y=w959:dbl)
            n528 = local write "TEC_current, mA"(w952) -> ()
            n529 = Absolute Value(x=w959) -> (abs(x)=w950:dbl)
            "IPD_ext, mA" <- w950
            n530 = local write "IPD(ext), mA"(w950) -> ()
            n531 = Multiply(x=w970, y=1000.0) -> (x*y=w951:dbl)
            "Operating Current" <- w951
            n532 = local write "Operating Current, mA"(w951) -> ()
          }
          frame #2 {
            n533 = Wait (ms)(milliseconds to wait=u32 100) -> ()  [unwired: 1 out]
          }
        }
      }
      frame True {
        n534 = Wait (ms)(milliseconds to wait=u32 20) -> ()  [unwired: 1 out]
      }
    }
  }
  n535 = while {
    tunnel: w4 -> [w986]
    tunnel: w1 -> [w985]
    stop <- FALSE stop-if-true
    n536 = local read "stop"() -> (w987:bool)
    n537 = case shown="True" w987 {
      tunnel: w986 -> [_ w990]
      tunnel: w985 -> [_ w989]
      frame False {
      }
      frame True {
        n538 = stacked-sequence {
          tunnel: w990 -> [_ _ _ _ w1009 _]
          tunnel: w989 -> [_ _ _ _ w1008 _]
          frame #0 {
            w991 = T1."Initialization"  # Case
            n539 = local write "Case"(w991) -> ()
          }
          frame #1 {
            # "Закрытие логов"
            n540 = property on="Op(Ild)_Log_address" class="Ref (strict)"() -> ("Value"=w995:refnum<file>)  [unwired: 2 in, 2 out]
            n541 = property on="Param_Log_address" class="Ref (strict)"() -> ("Value"=w996:refnum<file>)  [unwired: 2 in, 2 out]
            n542 = property on="V2(Ild)_Log_address" class="Ref (strict)"() -> ("Value"=w994:refnum<file>)  [unwired: 2 in, 2 out]
            n543 = Format Into String(initial string=w995, "\r\n") -> (resulting string=w1005:refnum<file>)  [unwired: 2 in, 1 out]
            n544 = Format Into String(initial string=w996, "\r\n") -> (resulting string=w1004:refnum<file>)  [unwired: 2 in, 1 out]
            n545 = Format Into String(initial string=w994, "\r\n") -> (resulting string=w1002:refnum<file>)  [unwired: 2 in, 1 out]
            n546 = Close File(refnum=w1005) -> ()  [unwired: 1 in, 2 out]
            n547 = Close File(refnum=w1004) -> ()  [unwired: 1 in, 2 out]
            n548 = Close File(refnum=w1002) -> ()  [unwired: 1 in, 2 out]
            n549 = property on="Ipd(Ild)_Monitor_Log_address" class="Ref (strict)"() -> ("Value"=w992:refnum<file>)  [unwired: 2 in, 2 out]
            n550 = property on="Ipd(Ild)_External_Log_address" class="Ref (strict)"() -> ("Value"=w993:refnum<file>)  [unwired: 2 in, 2 out]
            n551 = Format Into String(initial string=w993, "\r\n") -> (resulting string=w999:refnum<file>)  [unwired: 2 in, 1 out]
            n552 = Format Into String(initial string=w992, "\r\n") -> (resulting string=w998:refnum<file>)  [unwired: 2 in, 1 out]
            n553 = Close File(refnum=w999) -> ()  [unwired: 1 in, 2 out]
            n554 = Close File(refnum=w998) -> ()  [unwired: 1 in, 2 out]
          }
          frame #2 {
            # "Выключение Офира"
          }
          frame #3 {
            w1007 = FALSE
            n555 = local write "Раб. режим LD"(w1007) -> ()
            n556 = local write "Хар-ки от I_LD"(w1007) -> ()
            n557 = local write "Power Enable"(w1007) -> ()
            n558 = local write "Хар-ка TEC"(w1007) -> ()
          }
          frame #4 {
            w1012 = "0,1,2" ("channel name")
            w1017 = "0,1,2" ("channel name")
            n559 = call <instrlib>:"niDCPower Configure Voltage Level.vi"("voltage level"=0.0, "channel name"=w1017, "instrument handle"=w1009) -> ("instrument handle out"=w1016:refnum<k15>)  [unwired: 7 in, 1 out]
            n560 = call <instrlib>:"niDCPower Configure Voltage Level.vi"("voltage level"=0.0, "channel name"=w1012, "instrument handle"=w1008) -> ("instrument handle out"=w1013:refnum<k15>)  [unwired: 7 in, 1 out]
            n561 = call <instrlib>:"niDCPower Configure Output Enabled.vi"("output enabled"=FALSE, "channel name"=w1017, "instrument handle"=w1016) -> ("instrument handle out"=w1015:refnum<k15>)  [unwired: 7 in, 1 out]
            n562 = call <instrlib>:"niDCPower Configure Output Enabled.vi"("output enabled"=FALSE, "channel name"=w1012, "instrument handle"=w1013) -> ("instrument handle out"=w1014:refnum<k15>)  [unwired: 7 in, 1 out]
            n563 = call <instrlib>:"niDCPower Close.vi"("instrument handle"=w1015) -> ()  [unwired: 10 in, 1 out]
            n564 = call <instrlib>:"niDCPower Close.vi"("instrument handle"=w1014) -> ()  [unwired: 10 in, 1 out]
          }
          frame #5 {
            n565 = Stop(stop? (T)=TRUE) -> ()
          }
        }
      }
    }
  }
  n566 = disable-structure shown="Disabled" {
    frame Disabled {
      n567 = local read "4070_address"() -> (w1024:refnum<k15>)
      n568 = local read "TEC_Source"() -> (w1021:enum16{"S1_Ch2", "S2_Ch0", "S3_Ch1"})
      n569 = case shown="\"S3_Ch1\"" w1021 {
        tunnel: [w1034 w1036 w1038] -> w1023
        tunnel: ["2" "0" "1"] -> w1022
        frame "S1_Ch2", Default {
          n570 = local read "Source_1_Vcc_out"() -> (w1034:refnum<k15>)
        }
        frame "S2_Ch0" {
          n571 = local read "Source_2_Vcc_out"() -> (w1036:refnum<k15>)
        }
        frame "S3_Ch1" {
          n572 = local read "Source_3_Vcc_out"() -> (w1038:refnum<k15>)
        }
      }
      n573 = call "Res_stabiliz.vi"("Точность ThRes"="Точность ThRes", "Up_Volt_limit"="the upper limit for the voltage", "Optimum ThRes"="Optimum ThRes", "Low_Volt_limit"="the lower limit for the voltage", "TEC_Source"=w1023, "4070_address"=w1024, "channel name"=w1022) -> ("Подстроенное напряжение"=→"Подстроенное напряжение\nстабилизации":dbl, "ThRes value"=→"ThRes value":dbl, "thRes_adj"=w1032:dbl, "Start Voltage"=w1025:dbl)  [unwired: 1 out]
      n574 = local write "Сопротивление терморез-ра"(w1032) -> ()
    }
    frame Enabled {
    }
  }
  n575 = disable-structure shown="Enabled" {
    frame Disabled {
      # "Есть в инициализации"
      # "Для измерения Сопротивления"
      # "Поменять in0/in1 для ТЕС"
      n576 = local read "Source_2_Vcc_out"() -> (w1044:refnum<k15>)
      n577 = local read "4070_Rele_source"() -> (w1039:enum16{"S2_Ch0", "S1_Ch2"})
      n578 = call <instrlib>:"niDCPower Configure Voltage Level.vi"("voltage level"=-5.0, "channel name"="2", "instrument handle"=w1044) -> ()  [unwired: 7 in, 2 out]
      n579 = case shown="\"S1_Ch2\"" w1039 {
        tunnel: [5.0 -5.0] -> w1040
        tunnel: ["0" "2"] -> w1041
        tunnel: [w1046 w1049] -> w1042
        frame "S2_Ch0", Default {
          n580 = local read "Source_2_Vcc_out"() -> (w1046:refnum<k15>)
        }
        frame "S1_Ch2" {
          n581 = local read "Source_1_Vcc_out"() -> (w1049:refnum<k15>)
        }
      }
      n582 = call <instrlib>:"niDCPower Configure Voltage Level.vi"("voltage level"=w1040, "channel name"=w1041, "instrument handle"=w1042) -> ()  [unwired: 7 in, 2 out]
    }
    frame Enabled {
    }
  }
  "Выполняется" <- w5
